vi "test json roundtrip.vi"(8 "error in (no error)":errorcluster, 11 "Enum":T1(ring)) -> (0 "error out":errorcluster, 1 "JSON out":string, 2 "JSON in":string, 3 "Passed?":bool, 5 "Result":variant)   [LabVIEW 2019, in "labview_json_tests.lvlib"]
uses:
  labview_json_tests.lvlib
  lib/labview_json.lvlib
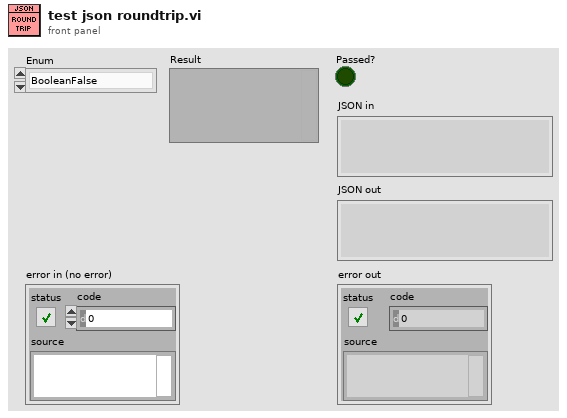
[diagram p1: front panel]
types:
  T1 = enum16{"BooleanFalse", "BooleanTrue", "StringSentence", "StringMultiline", "StringQuoted", "StringEscaped", "IntNumber", "IntMin", "IntMax", "IntI64", "IntI32", "IntI16", "IntI8", "UintNumber", "UintMin", "UintMax", "UintU64", "UintU32", "UintU16", "UintU8", "FloatNumber", "FloatMin", "FloatMax", "FloatZero", "FloatNaN", "FloatExt", "FloatDbl", "FloatSgl", "EnumU32", "EnumU16", "EnumU8", "EnumU32String", "EnumU16String", "EnumU8String", "EnumBadString", "PathAbs", "PathRel", "PathNetwork", "PathFile", "PathEmpty", "PathNaN", "PathCurrentDir", "PathParentDir", "TimeDateTime", "TimeDate", "NullVoid", "NullLVVariant", "NullBoolean", "NullInt", "NullUint", "NullFloat", "NullString", "NullPath", "NullEnum", "NullTime", "NullArray", "NullArrayVoid", "NullArrayLVVariant", "NullObject", "NullObjectVoid", "NullObjectLVVariant", "NullWaveform", "Array1DValues", "Array1DEmpty", "Array1DObject", "Array1DMulti", "Array2DValues", "Array2DEmpty", "Array3DValues", "Array3DEmpty", "ObjectValues", "ObjectEmpty", "ObjectWaveform", "ObjectReorder"}
  T2 = cluster{"I16":i16, "Bool":bool, "String":string, "Array":u32[]}
  T3 = enum16{"Item A", "Item B", "Item C", "Item D", "Item E"}
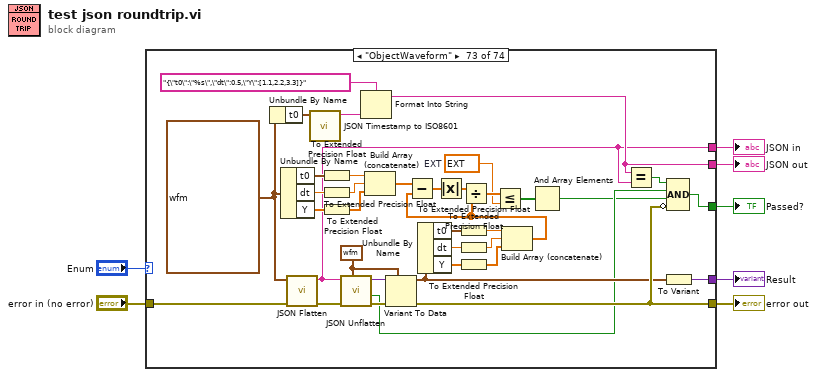
[diagram p0: block diagram]
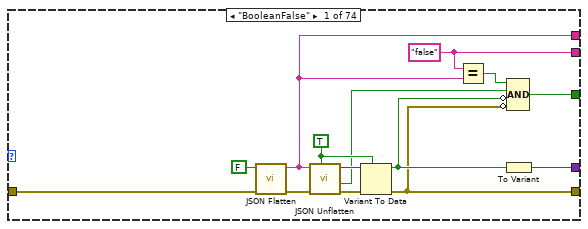
[diagram p2: hidden frame]
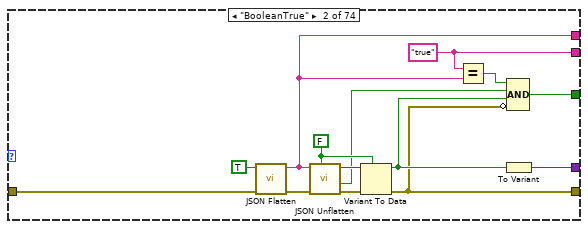
[diagram p3: hidden frame]
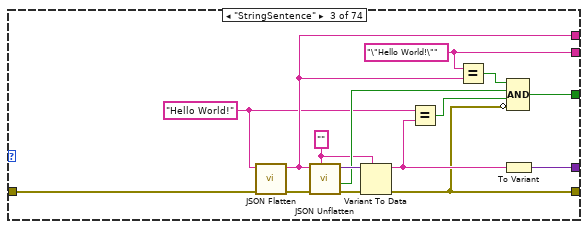
[diagram p4: hidden frame]
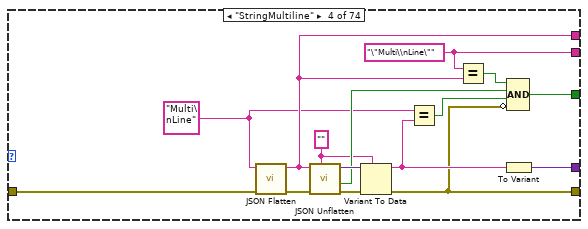
[diagram p5: hidden frame]
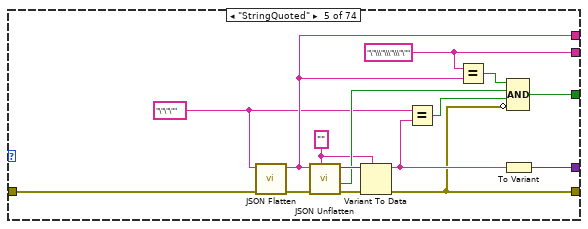
[diagram p6: hidden frame]
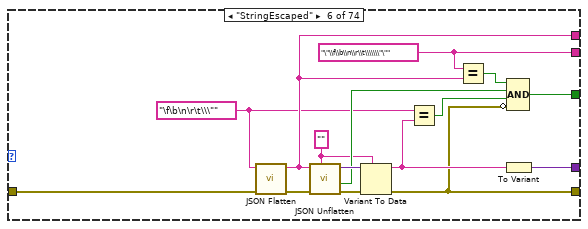
[diagram p7: hidden frame]
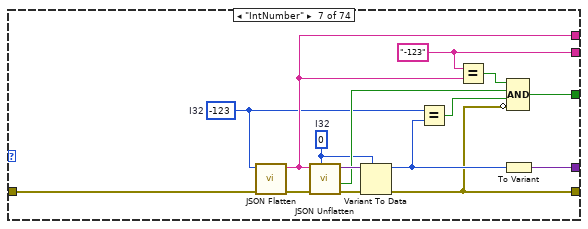
[diagram p8: hidden frame]
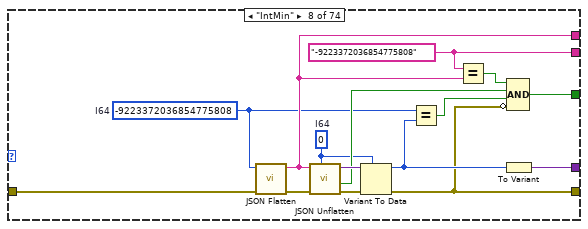
[diagram p9: hidden frame]
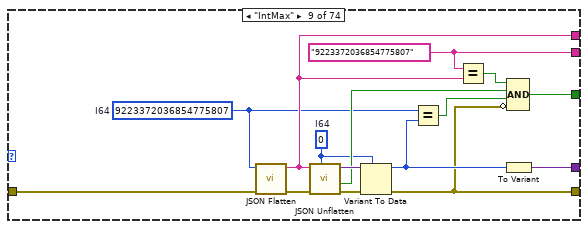
[diagram p10: hidden frame]
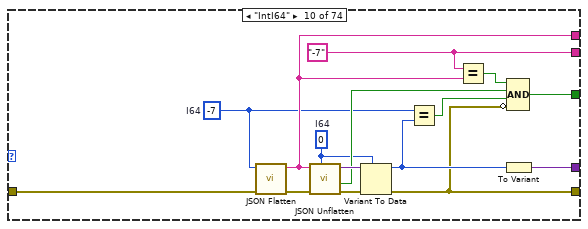
[diagram p11: hidden frame]
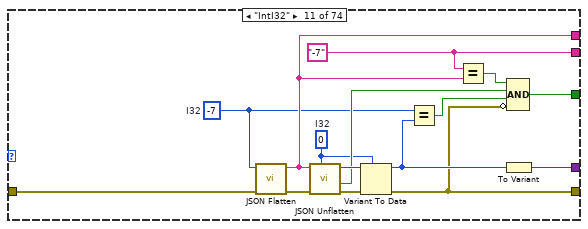
[diagram p12: hidden frame]
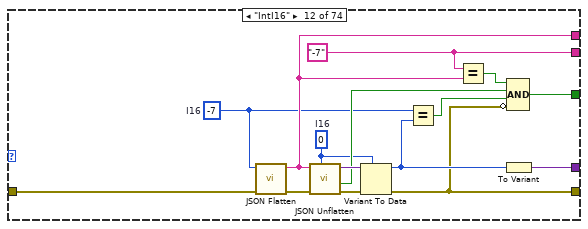
[diagram p13: hidden frame]
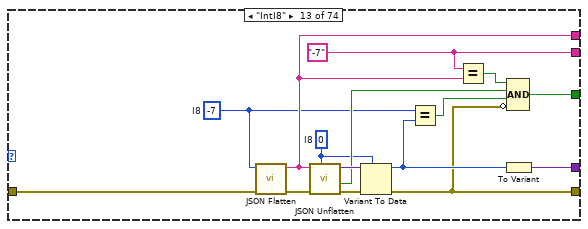
[diagram p14: hidden frame]
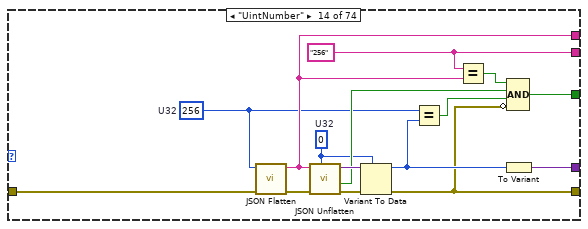
[diagram p15: hidden frame]
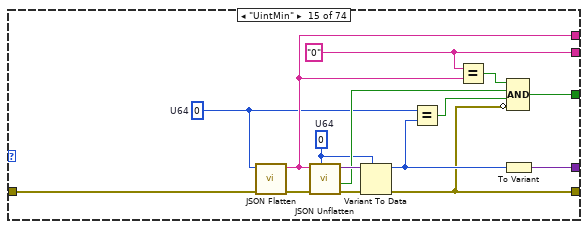
[diagram p16: hidden frame]
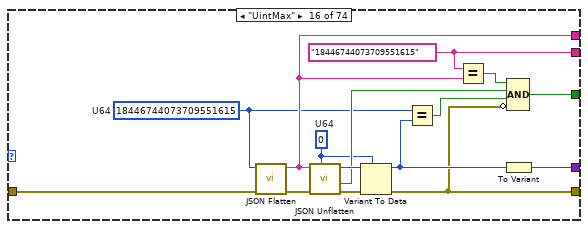
[diagram p17: hidden frame]
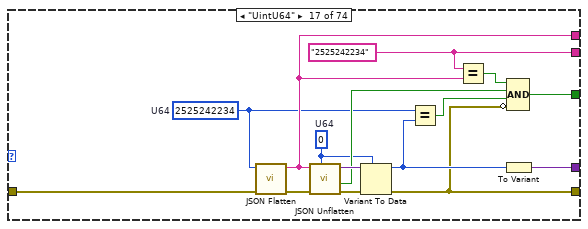
[diagram p18: hidden frame]
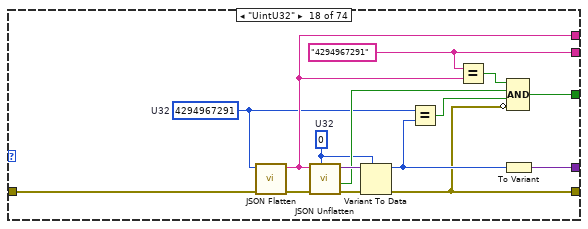
[diagram p19: hidden frame]
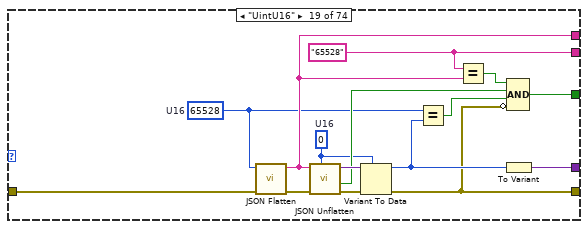
[diagram p20: hidden frame]
diagram:
  n1 = case shown="\"ObjectWaveform\"" "Enum" {
    tunnel: "error in (no error)" -> [w17 w31 w46 w61 w76 w91 w106 w121 w136 w151 w166 w181 w196 w211 w226 w241 w256 w271 w286 w301 w320 w335 w350 w365 w380 w399 w418 w437 w453 w469 w485 w501 w517 w533 w549 w564 w579 w594 w609 w624 w639 w654 w669 w694 w702 w731 w750 w758 w771 w784 w797 w810 w822 w835 w848 w862 w873 w887 w901 w914 w929 w942 w961 w977 w992 w1024 w1040 w1056 w1072 w1088 w1105 w1122 w1159 w1179]
    tunnel: [w8 w22 w36 w51 w66 w81 w96 w111 w126 w141 w156 w171 w186 w201 w216 w231 w246 w261 w276 w291 w306 w325 w340 w355 w370 w385 w404 w423 w442 w458 w474 w490 w506 w522 w539 w554 w569 w584 w599 w614 w629 w644 w659 w688 w713 w725 w740 w759 w772 w785 w798 w811 w823 w836 w849 w863 w875 w889 w902 w915 w930 w943 w951 w967 w986 w1019 w1030 w1046 w1062 w1078 w1099 w1116 w1156 w1173] -> w6
    tunnel: [w20 w34 w49 w64 w79 w94 w109 w124 w139 w154 w169 w184 w199 w214 w229 w244 w259 w274 w289 w304 w323 w338 w353 w368 w383 w402 w421 w440 w456 w472 w488 w504 w520 w536 w552 w567 w582 w597 w612 w627 w642 w657 w672 w697 w719 w734 w753 w764 w777 w790 w803 w816 w828 w841 w854 w868 w880 w894 w907 w920 w935 w948 w964 w980 w995 w1027 w1043 w1059 w1075 w1091 w1108 w1125 w1162 w1182] -> w5
    tunnel: [w19 w33 w48 w63 w78 w93 w108 w123 w138 w153 w168 w183 w198 w213 w228 w243 w258 w273 w288 w303 w322 w337 w352 w367 w382 w401 w420 w439 w455 w471 w487 w503 w519 w535 w551 w566 w581 w596 w611 w626 w641 w656 w671 w696 w718 w733 w752 w763 w776 w789 w802 w815 w827 w840 w853 w867 w879 w893 w906 w919 w934 w947 w963 w979 w994 w1026 w1042 w1058 w1074 w1090 w1107 w1124 w1161 w1181] -> w4
    tunnel: [w9 w23 w41 w56 w71 w82 w99 w114 w129 w144 w159 w174 w189 w204 w219 w234 w249 w264 w279 w294 w315 w330 w345 w360 w375 w394 w413 w432 w446 w462 w478 w494 w510 w526 w543 w557 w572 w587 w602 w617 w632 w647 w662 w676 w699 w728 w747 w755 w770 w783 w796 w809 w821 w834 w847 w861 w874 w888 w900 w913 w928 w941 w954 w970 w984 w1018 w1033 w1049 w1065 w1081 w1100 w1117 w1151 w1174] -> w2
    tunnel: [w15 w29 w44 w59 w74 w89 w104 w119 w134 w149 w164 w179 w194 w209 w224 w239 w254 w269 w284 w299 w318 w333 w348 w363 w378 w397 w416 w435 w451 w467 w483 w499 w515 w531 w547 w562 w577 w592 w607 w622 w637 w652 w667 w692 w699 w730 w749 w755 w770 w783 w796 w809 w821 w834 w847 w861 w874 w888 w900 w913 w928 w941 w959 w975 w990 w1022 w1038 w1054 w1070 w1086 w1103 w1120 w1132 w1177] -> w1
    frame "BooleanFalse" {
      w9 = "false"
      w12 = TRUE
      n2 = call "JSON Flatten.vi"("error in (no error)"=w17, "Variant in"=FALSE) -> ("error out"=w18:errorcluster, "JSON out"=w15:string)  [unwired: 8 in]
      n3 = call "JSON Unflatten.vi"("Variant Type"=w12, "error in (no error)"=w18, "JSON in"=w15) -> ("error out"=w16:errorcluster, "Exists?"=w11:bool, "Variant out"=w13:variant)  [unwired: 6 in]
      n4 = Variant To Data(error in=w16, type=w12, Variant=w13) -> (data=w10:bool, error out=w8:errorcluster)
      n5 = Equal?(x=w9, y=w15) -> (x = y?=w21:bool)
      n6 = To Variant(anything=w10) -> (Variant=w19:variant)
      n7 = Compound Arithmetic op=AND(w21, w11, invert w10, invert w8) -> (w20:bool)
    }
    frame "BooleanTrue" {
      w23 = "true"
      w26 = FALSE
      n8 = call "JSON Flatten.vi"("error in (no error)"=w31, "Variant in"=TRUE) -> ("error out"=w32:errorcluster, "JSON out"=w29:string)  [unwired: 8 in]
      n9 = call "JSON Unflatten.vi"("Variant Type"=w26, "error in (no error)"=w32, "JSON in"=w29) -> ("error out"=w30:errorcluster, "Exists?"=w25:bool, "Variant out"=w27:variant)  [unwired: 6 in]
      n10 = Variant To Data(error in=w30, type=w26, Variant=w27) -> (data=w24:bool, error out=w22:errorcluster)
      n11 = Equal?(x=w23, y=w29) -> (x = y?=w35:bool)
      n12 = To Variant(anything=w24) -> (Variant=w33:variant)
      n13 = Compound Arithmetic op=AND(w35, w25, w24, invert w22) -> (w34:bool)
    }
    frame "StringSentence" {
      w40 = ""
      w38 = "Hello World!"
      w41 = "\"Hello World!\""
      n14 = call "JSON Flatten.vi"("error in (no error)"=w46, "Variant in"=w38) -> ("error out"=w47:errorcluster, "JSON out"=w44:string)  [unwired: 8 in]
      n15 = call "JSON Unflatten.vi"("Variant Type"=w40, "error in (no error)"=w47, "JSON in"=w44) -> ("error out"=w45:errorcluster, "Exists?"=w42:bool, "Variant out"=w43:variant)  [unwired: 6 in]
      n16 = Variant To Data(error in=w45, type=w40, Variant=w43) -> (data=w39:string, error out=w36:errorcluster)
      n17 = Equal?(x=w38, y=w39) -> (x = y?=w37:bool)
      n18 = Equal?(x=w41, y=w44) -> (x = y?=w50:bool)
      n19 = To Variant(anything=w39) -> (Variant=w48:variant)
      n20 = Compound Arithmetic op=AND(w50, w42, w37, invert w36) -> (w49:bool)
    }
    frame "StringMultiline" {
      w55 = ""
      w53 = "Multi\nLine"
      w56 = "\"Multi\\nLine\""
      n21 = call "JSON Flatten.vi"("error in (no error)"=w61, "Variant in"=w53) -> ("error out"=w62:errorcluster, "JSON out"=w59:string)  [unwired: 8 in]
      n22 = call "JSON Unflatten.vi"("Variant Type"=w55, "error in (no error)"=w62, "JSON in"=w59) -> ("error out"=w60:errorcluster, "Exists?"=w57:bool, "Variant out"=w58:variant)  [unwired: 6 in]
      n23 = Variant To Data(error in=w60, type=w55, Variant=w58) -> (data=w54:string, error out=w51:errorcluster)
      n24 = Equal?(x=w53, y=w54) -> (x = y?=w52:bool)
      n25 = Equal?(x=w56, y=w59) -> (x = y?=w65:bool)
      n26 = To Variant(anything=w54) -> (Variant=w63:variant)
      n27 = Compound Arithmetic op=AND(w65, w57, w52, invert w51) -> (w64:bool)
    }
    frame "StringQuoted" {
      w70 = ""
      w68 = "\"\"\""
      w71 = "\"\\\"\\\"\\\"\""
      n28 = call "JSON Flatten.vi"("error in (no error)"=w76, "Variant in"=w68) -> ("error out"=w77:errorcluster, "JSON out"=w74:string)  [unwired: 8 in]
      n29 = call "JSON Unflatten.vi"("Variant Type"=w70, "error in (no error)"=w77, "JSON in"=w74) -> ("error out"=w75:errorcluster, "Exists?"=w72:bool, "Variant out"=w73:variant)  [unwired: 6 in]
      n30 = Variant To Data(error in=w75, type=w70, Variant=w73) -> (data=w69:string, error out=w66:errorcluster)
      n31 = Equal?(x=w68, y=w69) -> (x = y?=w67:bool)
      n32 = Equal?(x=w71, y=w74) -> (x = y?=w80:bool)
      n33 = To Variant(anything=w69) -> (Variant=w78:variant)
      n34 = Compound Arithmetic op=AND(w80, w72, w67, invert w66) -> (w79:bool)
    }
    frame "StringEscaped" {
      w83 = "\f\b\n\r\t\\\""
      w82 = "\"\\f\\b\\n\\r\\t\\\\\\\"\""
      w86 = ""
      n35 = call "JSON Flatten.vi"("error in (no error)"=w91, "Variant in"=w83) -> ("error out"=w92:errorcluster, "JSON out"=w89:string)  [unwired: 8 in]
      n36 = call "JSON Unflatten.vi"("Variant Type"=w86, "error in (no error)"=w92, "JSON in"=w89) -> ("error out"=w90:errorcluster, "Exists?"=w87:bool, "Variant out"=w88:variant)  [unwired: 6 in]
      n37 = Variant To Data(error in=w90, type=w86, Variant=w88) -> (data=w85:string, error out=w81:errorcluster)
      n38 = Equal?(x=w83, y=w85) -> (x = y?=w84:bool)
      n39 = Equal?(x=w82, y=w89) -> (x = y?=w95:bool)
      n40 = To Variant(anything=w85) -> (Variant=w93:variant)
      n41 = Compound Arithmetic op=AND(w95, w87, w84, invert w81) -> (w94:bool)
    }
    frame "IntNumber" {
      w97 = 0  # I32
      w98 = -123  # I32
      w99 = "-123"
      n42 = call "JSON Flatten.vi"("error in (no error)"=w106, "Variant in"=w98) -> ("error out"=w107:errorcluster, "JSON out"=w104:string)  [unwired: 8 in]
      n43 = call "JSON Unflatten.vi"("Variant Type"=w97, "error in (no error)"=w107, "JSON in"=w104) -> ("error out"=w105:errorcluster, "Exists?"=w102:bool, "Variant out"=w103:variant)  [unwired: 6 in]
      n44 = Variant To Data(error in=w105, type=w97, Variant=w103) -> (data=w101:i32, error out=w96:errorcluster)
      n45 = Equal?(x=w98, y=w101) -> (x = y?=w100:bool)
      n46 = Equal?(x=w99, y=w104) -> (x = y?=w110:bool)
      n47 = To Variant(anything=w101) -> (Variant=w108:variant)
      n48 = Compound Arithmetic op=AND(w110, w102, w100, invert w96) -> (w109:bool)
    }
    frame "IntMin" {
      w112 = i64 0  # I64
      w113 = i64 -9223372036854775808  # I64
      w114 = "-9223372036854775808"
      n49 = call "JSON Flatten.vi"("error in (no error)"=w121, "Variant in"=w113) -> ("error out"=w122:errorcluster, "JSON out"=w119:string)  [unwired: 8 in]
      n50 = call "JSON Unflatten.vi"("Variant Type"=w112, "error in (no error)"=w122, "JSON in"=w119) -> ("error out"=w120:errorcluster, "Exists?"=w117:bool, "Variant out"=w118:variant)  [unwired: 6 in]
      n51 = Variant To Data(error in=w120, type=w112, Variant=w118) -> (data=w116:i64, error out=w111:errorcluster)
      n52 = Equal?(x=w113, y=w116) -> (x = y?=w115:bool)
      n53 = Equal?(x=w114, y=w119) -> (x = y?=w125:bool)
      n54 = To Variant(anything=w116) -> (Variant=w123:variant)
      n55 = Compound Arithmetic op=AND(w125, w117, w115, invert w111) -> (w124:bool)
    }
    frame "IntMax" {
      w127 = i64 0  # I64
      w128 = i64 9223372036854775807  # I64
      w129 = "9223372036854775807"
      n56 = call "JSON Flatten.vi"("error in (no error)"=w136, "Variant in"=w128) -> ("error out"=w137:errorcluster, "JSON out"=w134:string)  [unwired: 8 in]
      n57 = call "JSON Unflatten.vi"("Variant Type"=w127, "error in (no error)"=w137, "JSON in"=w134) -> ("error out"=w135:errorcluster, "Exists?"=w132:bool, "Variant out"=w133:variant)  [unwired: 6 in]
      n58 = Variant To Data(error in=w135, type=w127, Variant=w133) -> (data=w131:i64, error out=w126:errorcluster)
      n59 = Equal?(x=w128, y=w131) -> (x = y?=w130:bool)
      n60 = Equal?(x=w129, y=w134) -> (x = y?=w140:bool)
      n61 = To Variant(anything=w131) -> (Variant=w138:variant)
      n62 = Compound Arithmetic op=AND(w140, w132, w130, invert w126) -> (w139:bool)
    }
    frame "IntI64" {
      w142 = i64 0  # I64
      w143 = i64 -7  # I64
      w144 = "-7"
      n63 = call "JSON Flatten.vi"("error in (no error)"=w151, "Variant in"=w143) -> ("error out"=w152:errorcluster, "JSON out"=w149:string)  [unwired: 8 in]
      n64 = call "JSON Unflatten.vi"("Variant Type"=w142, "error in (no error)"=w152, "JSON in"=w149) -> ("error out"=w150:errorcluster, "Exists?"=w147:bool, "Variant out"=w148:variant)  [unwired: 6 in]
      n65 = Variant To Data(error in=w150, type=w142, Variant=w148) -> (data=w146:i64, error out=w141:errorcluster)
      n66 = Equal?(x=w143, y=w146) -> (x = y?=w145:bool)
      n67 = Equal?(x=w144, y=w149) -> (x = y?=w155:bool)
      n68 = To Variant(anything=w146) -> (Variant=w153:variant)
      n69 = Compound Arithmetic op=AND(w155, w147, w145, invert w141) -> (w154:bool)
    }
    frame "IntI32" {
      w157 = 0  # I32
      w158 = -7  # I32
      w159 = "-7"
      n70 = call "JSON Flatten.vi"("error in (no error)"=w166, "Variant in"=w158) -> ("error out"=w167:errorcluster, "JSON out"=w164:string)  [unwired: 8 in]
      n71 = call "JSON Unflatten.vi"("Variant Type"=w157, "error in (no error)"=w167, "JSON in"=w164) -> ("error out"=w165:errorcluster, "Exists?"=w162:bool, "Variant out"=w163:variant)  [unwired: 6 in]
      n72 = Variant To Data(error in=w165, type=w157, Variant=w163) -> (data=w161:i32, error out=w156:errorcluster)
      n73 = Equal?(x=w158, y=w161) -> (x = y?=w160:bool)
      n74 = Equal?(x=w159, y=w164) -> (x = y?=w170:bool)
      n75 = To Variant(anything=w161) -> (Variant=w168:variant)
      n76 = Compound Arithmetic op=AND(w170, w162, w160, invert w156) -> (w169:bool)
    }
    frame "IntI16" {
      w172 = i16 0  # I16
      w173 = i16 -7  # I16
      w174 = "-7"
      n77 = call "JSON Flatten.vi"("error in (no error)"=w181, "Variant in"=w173) -> ("error out"=w182:errorcluster, "JSON out"=w179:string)  [unwired: 8 in]
      n78 = call "JSON Unflatten.vi"("Variant Type"=w172, "error in (no error)"=w182, "JSON in"=w179) -> ("error out"=w180:errorcluster, "Exists?"=w177:bool, "Variant out"=w178:variant)  [unwired: 6 in]
      n79 = Variant To Data(error in=w180, type=w172, Variant=w178) -> (data=w176:i16, error out=w171:errorcluster)
      n80 = Equal?(x=w173, y=w176) -> (x = y?=w175:bool)
      n81 = Equal?(x=w174, y=w179) -> (x = y?=w185:bool)
      n82 = To Variant(anything=w176) -> (Variant=w183:variant)
      n83 = Compound Arithmetic op=AND(w185, w177, w175, invert w171) -> (w184:bool)
    }
    frame "IntI8" {
      w187 = i8 0  # I8
      w188 = i8 -7  # I8
      w189 = "-7"
      n84 = call "JSON Flatten.vi"("error in (no error)"=w196, "Variant in"=w188) -> ("error out"=w197:errorcluster, "JSON out"=w194:string)  [unwired: 8 in]
      n85 = call "JSON Unflatten.vi"("Variant Type"=w187, "error in (no error)"=w197, "JSON in"=w194) -> ("error out"=w195:errorcluster, "Exists?"=w192:bool, "Variant out"=w193:variant)  [unwired: 6 in]
      n86 = Variant To Data(error in=w195, type=w187, Variant=w193) -> (data=w191:i8, error out=w186:errorcluster)
      n87 = Equal?(x=w188, y=w191) -> (x = y?=w190:bool)
      n88 = Equal?(x=w189, y=w194) -> (x = y?=w200:bool)
      n89 = To Variant(anything=w191) -> (Variant=w198:variant)
      n90 = Compound Arithmetic op=AND(w200, w192, w190, invert w186) -> (w199:bool)
    }
    frame "UintNumber" {
      w202 = u32 0  # U32
      w203 = u32 256  # U32
      w204 = "256"
      n91 = call "JSON Flatten.vi"("error in (no error)"=w211, "Variant in"=w203) -> ("error out"=w212:errorcluster, "JSON out"=w209:string)  [unwired: 8 in]
      n92 = call "JSON Unflatten.vi"("Variant Type"=w202, "error in (no error)"=w212, "JSON in"=w209) -> ("error out"=w210:errorcluster, "Exists?"=w207:bool, "Variant out"=w208:variant)  [unwired: 6 in]
      n93 = Variant To Data(error in=w210, type=w202, Variant=w208) -> (data=w206:u32, error out=w201:errorcluster)
      n94 = Equal?(x=w203, y=w206) -> (x = y?=w205:bool)
      n95 = Equal?(x=w204, y=w209) -> (x = y?=w215:bool)
      n96 = To Variant(anything=w206) -> (Variant=w213:variant)
      n97 = Compound Arithmetic op=AND(w215, w207, w205, invert w201) -> (w214:bool)
    }
    frame "UintMin" {
      w217 = u64 0  # U64
      w218 = u64 0  # U64
      w219 = "0"
      n98 = call "JSON Flatten.vi"("error in (no error)"=w226, "Variant in"=w218) -> ("error out"=w227:errorcluster, "JSON out"=w224:string)  [unwired: 8 in]
      n99 = call "JSON Unflatten.vi"("Variant Type"=w217, "error in (no error)"=w227, "JSON in"=w224) -> ("error out"=w225:errorcluster, "Exists?"=w222:bool, "Variant out"=w223:variant)  [unwired: 6 in]
      n100 = Variant To Data(error in=w225, type=w217, Variant=w223) -> (data=w221:u64, error out=w216:errorcluster)
      n101 = Equal?(x=w218, y=w221) -> (x = y?=w220:bool)
      n102 = Equal?(x=w219, y=w224) -> (x = y?=w230:bool)
      n103 = To Variant(anything=w221) -> (Variant=w228:variant)
      n104 = Compound Arithmetic op=AND(w230, w222, w220, invert w216) -> (w229:bool)
    }
    frame "UintMax" {
      w232 = u64 0  # U64
      w233 = u64 18446744073709551615  # U64
      w234 = "18446744073709551615"
      n105 = call "JSON Flatten.vi"("error in (no error)"=w241, "Variant in"=w233) -> ("error out"=w242:errorcluster, "JSON out"=w239:string)  [unwired: 8 in]
      n106 = call "JSON Unflatten.vi"("Variant Type"=w232, "error in (no error)"=w242, "JSON in"=w239) -> ("error out"=w240:errorcluster, "Exists?"=w237:bool, "Variant out"=w238:variant)  [unwired: 6 in]
      n107 = Variant To Data(error in=w240, type=w232, Variant=w238) -> (data=w236:u64, error out=w231:errorcluster)
      n108 = Equal?(x=w233, y=w236) -> (x = y?=w235:bool)
      n109 = Equal?(x=w234, y=w239) -> (x = y?=w245:bool)
      n110 = To Variant(anything=w236) -> (Variant=w243:variant)
      n111 = Compound Arithmetic op=AND(w245, w237, w235, invert w231) -> (w244:bool)
    }
    frame "UintU64" {
      w247 = u64 0  # U64
      w248 = u64 2525242234  # U64
      w249 = "2525242234"
      n112 = call "JSON Flatten.vi"("error in (no error)"=w256, "Variant in"=w248) -> ("error out"=w257:errorcluster, "JSON out"=w254:string)  [unwired: 8 in]
      n113 = call "JSON Unflatten.vi"("Variant Type"=w247, "error in (no error)"=w257, "JSON in"=w254) -> ("error out"=w255:errorcluster, "Exists?"=w252:bool, "Variant out"=w253:variant)  [unwired: 6 in]
      n114 = Variant To Data(error in=w255, type=w247, Variant=w253) -> (data=w251:u64, error out=w246:errorcluster)
      n115 = Equal?(x=w248, y=w251) -> (x = y?=w250:bool)
      n116 = Equal?(x=w249, y=w254) -> (x = y?=w260:bool)
      n117 = To Variant(anything=w251) -> (Variant=w258:variant)
      n118 = Compound Arithmetic op=AND(w260, w252, w250, invert w246) -> (w259:bool)
    }
    frame "UintU32" {
      w262 = u32 0  # U32
      w263 = u32 4294967291  # U32
      w264 = "4294967291"
      n119 = call "JSON Flatten.vi"("error in (no error)"=w271, "Variant in"=w263) -> ("error out"=w272:errorcluster, "JSON out"=w269:string)  [unwired: 8 in]
      n120 = call "JSON Unflatten.vi"("Variant Type"=w262, "error in (no error)"=w272, "JSON in"=w269) -> ("error out"=w270:errorcluster, "Exists?"=w267:bool, "Variant out"=w268:variant)  [unwired: 6 in]
      n121 = Variant To Data(error in=w270, type=w262, Variant=w268) -> (data=w266:u32, error out=w261:errorcluster)
      n122 = Equal?(x=w263, y=w266) -> (x = y?=w265:bool)
      n123 = Equal?(x=w264, y=w269) -> (x = y?=w275:bool)
      n124 = To Variant(anything=w266) -> (Variant=w273:variant)
      n125 = Compound Arithmetic op=AND(w275, w267, w265, invert w261) -> (w274:bool)
    }
    frame "UintU16" {
      w277 = u16 0  # U16
      w278 = u16 65528  # U16
      w279 = "65528"
      n126 = call "JSON Flatten.vi"("error in (no error)"=w286, "Variant in"=w278) -> ("error out"=w287:errorcluster, "JSON out"=w284:string)  [unwired: 8 in]
      n127 = call "JSON Unflatten.vi"("Variant Type"=w277, "error in (no error)"=w287, "JSON in"=w284) -> ("error out"=w285:errorcluster, "Exists?"=w282:bool, "Variant out"=w283:variant)  [unwired: 6 in]
      n128 = Variant To Data(error in=w285, type=w277, Variant=w283) -> (data=w281:u16, error out=w276:errorcluster)
      n129 = Equal?(x=w278, y=w281) -> (x = y?=w280:bool)
      n130 = Equal?(x=w279, y=w284) -> (x = y?=w290:bool)
      n131 = To Variant(anything=w281) -> (Variant=w288:variant)
      n132 = Compound Arithmetic op=AND(w290, w282, w280, invert w276) -> (w289:bool)
    }
    frame "UintU8" {
      w292 = u8 0  # U8
      w293 = u8 248  # U8
      w294 = "248"
      n133 = call "JSON Flatten.vi"("error in (no error)"=w301, "Variant in"=w293) -> ("error out"=w302:errorcluster, "JSON out"=w299:string)  [unwired: 8 in]
      n134 = call "JSON Unflatten.vi"("Variant Type"=w292, "error in (no error)"=w302, "JSON in"=w299) -> ("error out"=w300:errorcluster, "Exists?"=w297:bool, "Variant out"=w298:variant)  [unwired: 6 in]
      n135 = Variant To Data(error in=w300, type=w292, Variant=w298) -> (data=w296:u8, error out=w291:errorcluster)
      n136 = Equal?(x=w293, y=w296) -> (x = y?=w295:bool)
      n137 = Equal?(x=w294, y=w299) -> (x = y?=w305:bool)
      n138 = To Variant(anything=w296) -> (Variant=w303:variant)
      n139 = Compound Arithmetic op=AND(w305, w297, w295, invert w291) -> (w304:bool)
    }
    frame "FloatNumber" {
      w314 = 0.0  # DBL
      w313 = -42949.67289234  # DBL
      w315 = "-42949.67289234"
      n140 = call "JSON Flatten.vi"("error in (no error)"=w320, "Variant in"=w313) -> ("error out"=w321:errorcluster, "JSON out"=w318:string)  [unwired: 8 in]
      n141 = call "JSON Unflatten.vi"("Variant Type"=w314, "error in (no error)"=w321, "JSON in"=w318) -> ("error out"=w319:errorcluster, "Exists?"=w316:bool, "Variant out"=w317:variant)  [unwired: 6 in]
      n142 = Variant To Data(error in=w319, type=w314, Variant=w317) -> (data=w310:dbl, error out=w306:errorcluster)
      n143 = Subtract(x=w313, y=w310) -> (x-y=w312:dbl)
      n144 = Absolute Value(x=w312) -> (abs(x)=w311:dbl)
      n145 = Divide(x=w311, y=w310) -> (x/y=w309:dbl)
      n146 = Equal?(x=w315, y=w318) -> (x = y?=w324:bool)
      n147 = Less Or Equal?(x=w309, y=1e-11) -> (x <= y?=w307:bool)
      n148 = To Variant(anything=w310) -> (Variant=w322:variant)
      n149 = Compound Arithmetic op=AND(w324, w316, w307, invert w306) -> (w323:bool)
    }
    frame "FloatMin" {
      w329 = 0.0  # DBL
      w328 = -inf  # DBL
      w330 = "-Infinity"
      n150 = call "JSON Flatten.vi"("error in (no error)"=w335, "Variant in"=w328) -> ("error out"=w336:errorcluster, "JSON out"=w333:string)  [unwired: 8 in]
      n151 = call "JSON Unflatten.vi"("Variant Type"=w329, "error in (no error)"=w336, "JSON in"=w333) -> ("error out"=w334:errorcluster, "Exists?"=w331:bool, "Variant out"=w332:variant)  [unwired: 6 in]
      n152 = Variant To Data(error in=w334, type=w329, Variant=w332) -> (data=w327:dbl, error out=w325:errorcluster)
      n153 = Equal?(x=w330, y=w333) -> (x = y?=w339:bool)
      n154 = Equal?(x=w328, y=w327) -> (x = y?=w326:bool)
      n155 = To Variant(anything=w327) -> (Variant=w337:variant)
      n156 = Compound Arithmetic op=AND(w339, w331, w326, invert w325) -> (w338:bool)
    }
    frame "FloatMax" {
      w344 = 0.0  # DBL
      w343 = inf  # DBL
      w345 = "Infinity"
      n157 = call "JSON Flatten.vi"("error in (no error)"=w350, "Variant in"=w343) -> ("error out"=w351:errorcluster, "JSON out"=w348:string)  [unwired: 8 in]
      n158 = call "JSON Unflatten.vi"("Variant Type"=w344, "error in (no error)"=w351, "JSON in"=w348) -> ("error out"=w349:errorcluster, "Exists?"=w346:bool, "Variant out"=w347:variant)  [unwired: 6 in]
      n159 = Variant To Data(error in=w349, type=w344, Variant=w347) -> (data=w342:dbl, error out=w340:errorcluster)
      n160 = Equal?(x=w345, y=w348) -> (x = y?=w354:bool)
      n161 = Equal?(x=w343, y=w342) -> (x = y?=w341:bool)
      n162 = To Variant(anything=w342) -> (Variant=w352:variant)
      n163 = Compound Arithmetic op=AND(w354, w346, w341, invert w340) -> (w353:bool)
    }
    frame "FloatZero" {
      w359 = 2.0  # DBL
      w358 = 0.0  # DBL
      w360 = "0"
      n164 = call "JSON Flatten.vi"("error in (no error)"=w365, "Variant in"=w358) -> ("error out"=w366:errorcluster, "JSON out"=w363:string)  [unwired: 8 in]
      n165 = call "JSON Unflatten.vi"("Variant Type"=w359, "error in (no error)"=w366, "JSON in"=w363) -> ("error out"=w364:errorcluster, "Exists?"=w361:bool, "Variant out"=w362:variant)  [unwired: 6 in]
      n166 = Variant To Data(error in=w364, type=w359, Variant=w362) -> (data=w357:dbl, error out=w355:errorcluster)
      n167 = Equal?(x=w360, y=w363) -> (x = y?=w369:bool)
      n168 = Equal?(x=w358, y=w357) -> (x = y?=w356:bool)
      n169 = To Variant(anything=w357) -> (Variant=w367:variant)
      n170 = Compound Arithmetic op=AND(w369, w361, w356, invert w355) -> (w368:bool)
    }
    frame "FloatNaN" {
      w374 = 2.0  # DBL
      w373 = nan  # DBL
      w375 = "NaN"
      n171 = call "JSON Flatten.vi"("error in (no error)"=w380, "Variant in"=w373) -> ("error out"=w381:errorcluster, "JSON out"=w378:string)  [unwired: 8 in]
      n172 = call "JSON Unflatten.vi"("Variant Type"=w374, "error in (no error)"=w381, "JSON in"=w378) -> ("error out"=w379:errorcluster, "Exists?"=w376:bool, "Variant out"=w377:variant)  [unwired: 6 in]
      n173 = Variant To Data(error in=w379, type=w374, Variant=w377) -> (data=w372:dbl, error out=w370:errorcluster)
      n174 = Not A Number/Path/Refnum?(number/path/refnum=w372) -> (NaN/Path/Refnum?=w371:bool)
      n175 = Equal?(x=w375, y=w378) -> (x = y?=w384:bool)
      n176 = To Variant(anything=w372) -> (Variant=w382:variant)
      n177 = Compound Arithmetic op=AND(w384, w376, w371, invert w370) -> (w383:bool)
    }
    frame "FloatExt" {
      w387 = ext 1e-13  # EXT
      w393 = ext 0.0  # EXT
      w392 = ext 1.844674407371e+19  # EXT
      w394 = "1.844674407371E+19"
      n178 = call "JSON Flatten.vi"("error in (no error)"=w399, "Variant in"=w392) -> ("error out"=w400:errorcluster, "JSON out"=w397:string)  [unwired: 8 in]
      n179 = call "JSON Unflatten.vi"("Variant Type"=w393, "error in (no error)"=w400, "JSON in"=w397) -> ("error out"=w398:errorcluster, "Exists?"=w395:bool, "Variant out"=w396:variant)  [unwired: 6 in]
      n180 = Variant To Data(error in=w398, type=w393, Variant=w396) -> (data=w389:ext, error out=w385:errorcluster)
      n181 = Subtract(x=w392, y=w389) -> (x-y=w391:ext)
      n182 = Absolute Value(x=w391) -> (abs(x)=w390:ext)
      n183 = Divide(x=w390, y=w389) -> (x/y=w388:ext)
      n184 = Equal?(x=w394, y=w397) -> (x = y?=w403:bool)
      n185 = Less Or Equal?(x=w388, y=w387) -> (x <= y?=w386:bool)
      n186 = To Variant(anything=w389) -> (Variant=w401:variant)
      n187 = Compound Arithmetic op=AND(w403, w395, w386, invert w385) -> (w402:bool)
    }
    frame "FloatDbl" {
      w406 = 1e-11  # DBL
      w412 = 0.0  # DBL
      w411 = -19273791.23844  # DBL
      w413 = "-19273791.2384399995"
      n188 = call "JSON Flatten.vi"("error in (no error)"=w418, "Variant in"=w411) -> ("error out"=w419:errorcluster, "JSON out"=w416:string)  [unwired: 8 in]
      n189 = call "JSON Unflatten.vi"("Variant Type"=w412, "error in (no error)"=w419, "JSON in"=w416) -> ("error out"=w417:errorcluster, "Exists?"=w414:bool, "Variant out"=w415:variant)  [unwired: 6 in]
      n190 = Variant To Data(error in=w417, type=w412, Variant=w415) -> (data=w408:dbl, error out=w404:errorcluster)
      n191 = Subtract(x=w411, y=w408) -> (x-y=w410:dbl)
      n192 = Absolute Value(x=w410) -> (abs(x)=w409:dbl)
      n193 = Divide(x=w409, y=w408) -> (x/y=w407:dbl)
      n194 = Equal?(x=w413, y=w416) -> (x = y?=w422:bool)
      n195 = Less Or Equal?(x=w407, y=w406) -> (x <= y?=w405:bool)
      n196 = To Variant(anything=w408) -> (Variant=w420:variant)
      n197 = Compound Arithmetic op=AND(w422, w414, w405, invert w404) -> (w421:bool)
    }
    frame "FloatSgl" {
      w425 = sgl 1e-05  # SGL
      w431 = sgl 0.0  # SGL
      w430 = sgl 82833.23  # SGL
      w432 = "82833.2265625"
      n198 = call "JSON Flatten.vi"("error in (no error)"=w437, "Variant in"=w430) -> ("error out"=w438:errorcluster, "JSON out"=w435:string)  [unwired: 8 in]
      n199 = call "JSON Unflatten.vi"("Variant Type"=w431, "error in (no error)"=w438, "JSON in"=w435) -> ("error out"=w436:errorcluster, "Exists?"=w433:bool, "Variant out"=w434:variant)  [unwired: 6 in]
      n200 = Variant To Data(error in=w436, type=w431, Variant=w434) -> (data=w427:sgl, error out=w423:errorcluster)
      n201 = Subtract(x=w430, y=w427) -> (x-y=w429:sgl)
      n202 = Absolute Value(x=w429) -> (abs(x)=w428:sgl)
      n203 = Divide(x=w428, y=w427) -> (x/y=w426:sgl)
      n204 = Equal?(x=w432, y=w435) -> (x = y?=w441:bool)
      n205 = Less Or Equal?(x=w426, y=w425) -> (x <= y?=w424:bool)
      n206 = To Variant(anything=w427) -> (Variant=w439:variant)
      n207 = Compound Arithmetic op=AND(w441, w433, w424, invert w423) -> (w440:bool)
    }
    frame "EnumU32" {
      w444 = enum32{"Item A", "Item B", "Item C", "Item D"}."Item A"  # U32
      w445 = enum32{"Item A", "Item B", "Item C", "Item D"}."Item C"  # U32
      w446 = "2"
      n208 = call "JSON Flatten.vi"("Enums as string? (F)"=FALSE, "error in (no error)"=w453, "Variant in"=w445) -> ("error out"=w454:errorcluster, "JSON out"=w451:string)  [unwired: 7 in]
      n209 = call "JSON Unflatten.vi"("Variant Type"=w444, "error in (no error)"=w454, "JSON in"=w451) -> ("error out"=w452:errorcluster, "Exists?"=w449:bool, "Variant out"=w450:variant)  [unwired: 6 in]
      n210 = Variant To Data(error in=w452, type=w444, Variant=w450) -> (data=w448:enum32{"Item A", "Item B", "Item C", "Item D"}, error out=w442:errorcluster)
      n211 = Equal?(x=w445, y=w448) -> (x = y?=w447:bool)
      n212 = Equal?(x=w446, y=w451) -> (x = y?=w457:bool)
      n213 = To Variant(anything=w448) -> (Variant=w455:variant)
      n214 = Compound Arithmetic op=AND(w457, w449, w447, invert w442) -> (w456:bool)
    }
    frame "EnumU16" {
      w460 = enum16{"Item A", "Item B", "Item C", "Item D"}."Item A"  # U16
      w461 = enum16{"Item A", "Item B", "Item C", "Item D"}."Item B"  # U16
      w462 = "1"
      n215 = call "JSON Flatten.vi"("Enums as string? (F)"=FALSE, "error in (no error)"=w469, "Variant in"=w461) -> ("error out"=w470:errorcluster, "JSON out"=w467:string)  [unwired: 7 in]
      n216 = call "JSON Unflatten.vi"("Variant Type"=w460, "error in (no error)"=w470, "JSON in"=w467) -> ("error out"=w468:errorcluster, "Exists?"=w465:bool, "Variant out"=w466:variant)  [unwired: 6 in]
      n217 = Variant To Data(error in=w468, type=w460, Variant=w466) -> (data=w464:enum16{"Item A", "Item B", "Item C", "Item D"}, error out=w458:errorcluster)
      n218 = Equal?(x=w461, y=w464) -> (x = y?=w463:bool)
      n219 = Equal?(x=w462, y=w467) -> (x = y?=w473:bool)
      n220 = To Variant(anything=w464) -> (Variant=w471:variant)
      n221 = Compound Arithmetic op=AND(w473, w465, w463, invert w458) -> (w472:bool)
    }
    frame "EnumU8" {
      w476 = enum8{"Item A", "Item B", "Item C", "Item D"}."Item A"  # U8
      w477 = enum8{"Item A", "Item B", "Item C", "Item D"}."Item C"  # U8
      w478 = "2"
      n222 = call "JSON Flatten.vi"("Enums as string? (F)"=FALSE, "error in (no error)"=w485, "Variant in"=w477) -> ("error out"=w486:errorcluster, "JSON out"=w483:string)  [unwired: 7 in]
      n223 = call "JSON Unflatten.vi"("Variant Type"=w476, "error in (no error)"=w486, "JSON in"=w483) -> ("error out"=w484:errorcluster, "Exists?"=w481:bool, "Variant out"=w482:variant)  [unwired: 6 in]
      n224 = Variant To Data(error in=w484, type=w476, Variant=w482) -> (data=w480:enum8{"Item A", "Item B", "Item C", "Item D"}, error out=w474:errorcluster)
      n225 = Equal?(x=w477, y=w480) -> (x = y?=w479:bool)
      n226 = Equal?(x=w478, y=w483) -> (x = y?=w489:bool)
      n227 = To Variant(anything=w480) -> (Variant=w487:variant)
      n228 = Compound Arithmetic op=AND(w489, w481, w479, invert w474) -> (w488:bool)
    }
    frame "EnumU32String" {
      w492 = enum32{"Item A", "Item B", "Item C", "Item D"}."Item A"  # U32
      w493 = enum32{"Item A", "Item B", "Item C", "Item D"}."Item C"  # U32
      w494 = "\"Item C\""
      n229 = call "JSON Flatten.vi"("Enums as string? (F)"=TRUE, "error in (no error)"=w501, "Variant in"=w493) -> ("error out"=w502:errorcluster, "JSON out"=w499:string)  [unwired: 7 in]
      n230 = call "JSON Unflatten.vi"("Variant Type"=w492, "error in (no error)"=w502, "JSON in"=w499) -> ("error out"=w500:errorcluster, "Exists?"=w497:bool, "Variant out"=w498:variant)  [unwired: 6 in]
      n231 = Variant To Data(error in=w500, type=w492, Variant=w498) -> (data=w496:enum32{"Item A", "Item B", "Item C", "Item D"}, error out=w490:errorcluster)
      n232 = Equal?(x=w493, y=w496) -> (x = y?=w495:bool)
      n233 = Equal?(x=w494, y=w499) -> (x = y?=w505:bool)
      n234 = To Variant(anything=w496) -> (Variant=w503:variant)
      n235 = Compound Arithmetic op=AND(w505, w497, w495, invert w490) -> (w504:bool)
    }
    frame "EnumU16String" {
      w508 = enum16{"Item A", "Item B", "Item C", "Item D"}."Item A"  # U16
      w509 = enum16{"Item A", "Item B", "Item C", "Item D"}."Item B"  # U16
      w510 = "\"Item B\""
      n236 = call "JSON Flatten.vi"("Enums as string? (F)"=TRUE, "error in (no error)"=w517, "Variant in"=w509) -> ("error out"=w518:errorcluster, "JSON out"=w515:string)  [unwired: 7 in]
      n237 = call "JSON Unflatten.vi"("Variant Type"=w508, "error in (no error)"=w518, "JSON in"=w515) -> ("error out"=w516:errorcluster, "Exists?"=w513:bool, "Variant out"=w514:variant)  [unwired: 6 in]
      n238 = Variant To Data(error in=w516, type=w508, Variant=w514) -> (data=w512:enum16{"Item A", "Item B", "Item C", "Item D"}, error out=w506:errorcluster)
      n239 = Equal?(x=w509, y=w512) -> (x = y?=w511:bool)
      n240 = Equal?(x=w510, y=w515) -> (x = y?=w521:bool)
      n241 = To Variant(anything=w512) -> (Variant=w519:variant)
      n242 = Compound Arithmetic op=AND(w521, w513, w511, invert w506) -> (w520:bool)
    }
    frame "EnumU8String" {
      w524 = enum8{"Item A", "Item B", "Item C", "Item D"}."Item A"  # U8
      w525 = enum8{"Item A", "Item B", "Item C", "Item D"}."Item C"  # U8
      w526 = "\"Item C\""
      n243 = call "JSON Flatten.vi"("Enums as string? (F)"=TRUE, "error in (no error)"=w533, "Variant in"=w525) -> ("error out"=w534:errorcluster, "JSON out"=w531:string)  [unwired: 7 in]
      n244 = call "JSON Unflatten.vi"("Variant Type"=w524, "error in (no error)"=w534, "JSON in"=w531) -> ("error out"=w532:errorcluster, "Exists?"=w529:bool, "Variant out"=w530:variant)  [unwired: 6 in]
      n245 = Variant To Data(error in=w532, type=w524, Variant=w530) -> (data=w528:enum8{"Item A", "Item B", "Item C", "Item D"}, error out=w522:errorcluster)
      n246 = Equal?(x=w525, y=w528) -> (x = y?=w527:bool)
      n247 = Equal?(x=w526, y=w531) -> (x = y?=w537:bool)
      n248 = To Variant(anything=w528) -> (Variant=w535:variant)
      n249 = Compound Arithmetic op=AND(w537, w529, w527, invert w522) -> (w536:bool)
    }
    frame "EnumBadString" {
      w541 = enum16{"Item A", "Item B", "Item C", "Item D"}."Item A"  # U16
      w542 = T3."Item E"  # U16
      w543 = "\"Item E\""
      n250 = call "JSON Flatten.vi"("Enums as string? (F)"=TRUE, "error in (no error)"=w549, "Variant in"=w542) -> ("error out"=w550:errorcluster, "JSON out"=w547:string)  [unwired: 7 in]
      n251 = call "JSON Unflatten.vi"("Variant Type"=w541, "error in (no error)"=w550, "JSON in"=w547) -> ("error out"=w548:errorcluster, "Exists?"=w545:bool, "Variant out"=w546:variant)  [unwired: 6 in]
      n252 = Variant To Data(error in=w548, type=w541, Variant=w546) -> (data=w544:enum16{"Item A", "Item B", "Item C", "Item D"}, error out=w538:errorcluster)
      n253 = Equal?(x=w543, y=w547) -> (x = y?=w553:bool)
      n254 = To Variant(anything=w544) -> (Variant=w551:variant)
      n255 = call <vilib>:"Clear Errors.vi"("error in (no error)"=w538) -> ("error out"=w539:errorcluster)  [unwired: 5 in, 1 out]
      n256 = Compound Arithmetic op=AND(w553, invert w545, w538) -> (w552:bool)
    }
    frame "PathAbs" {
      w555 = path ""
      w556 = path "C:/"
      w557 = "\"C:\\\\\""
      n257 = call "JSON Flatten.vi"("error in (no error)"=w564, "Variant in"=w556) -> ("error out"=w565:errorcluster, "JSON out"=w562:string)  [unwired: 8 in]
      n258 = call "JSON Unflatten.vi"("Variant Type"=w555, "error in (no error)"=w565, "JSON in"=w562) -> ("error out"=w563:errorcluster, "Exists?"=w560:bool, "Variant out"=w561:variant)  [unwired: 6 in]
      n259 = Variant To Data(error in=w563, type=w555, Variant=w561) -> (data=w559:path, error out=w554:errorcluster)
      n260 = Equal?(x=w556, y=w559) -> (x = y?=w558:bool)
      n261 = Equal?(x=w557, y=w562) -> (x = y?=w568:bool)
      n262 = To Variant(anything=w559) -> (Variant=w566:variant)
      n263 = Compound Arithmetic op=AND(w568, w560, w558, invert w554) -> (w567:bool)
    }
    frame "PathRel" {
      w570 = path ""
      w571 = path "abc/def.txt"
      w572 = "\"abc\\\\def.txt\""
      n264 = call "JSON Flatten.vi"("error in (no error)"=w579, "Variant in"=w571) -> ("error out"=w580:errorcluster, "JSON out"=w577:string)  [unwired: 8 in]
      n265 = call "JSON Unflatten.vi"("Variant Type"=w570, "error in (no error)"=w580, "JSON in"=w577) -> ("error out"=w578:errorcluster, "Exists?"=w575:bool, "Variant out"=w576:variant)  [unwired: 6 in]
      n266 = Variant To Data(error in=w578, type=w570, Variant=w576) -> (data=w574:path, error out=w569:errorcluster)
      n267 = Equal?(x=w571, y=w574) -> (x = y?=w573:bool)
      n268 = Equal?(x=w572, y=w577) -> (x = y?=w583:bool)
      n269 = To Variant(anything=w574) -> (Variant=w581:variant)
      n270 = Compound Arithmetic op=AND(w583, w575, w573, invert w569) -> (w582:bool)
    }
    frame "PathNetwork" {
      w585 = path ""
      w586 = path "\\\\server\\folder"
      w587 = "\"\\\\\\\\server\\\\folder\""
      n271 = call "JSON Flatten.vi"("error in (no error)"=w594, "Variant in"=w586) -> ("error out"=w595:errorcluster, "JSON out"=w592:string)  [unwired: 8 in]
      n272 = call "JSON Unflatten.vi"("Variant Type"=w585, "error in (no error)"=w595, "JSON in"=w592) -> ("error out"=w593:errorcluster, "Exists?"=w590:bool, "Variant out"=w591:variant)  [unwired: 6 in]
      n273 = Variant To Data(error in=w593, type=w585, Variant=w591) -> (data=w589:path, error out=w584:errorcluster)
      n274 = Equal?(x=w586, y=w589) -> (x = y?=w588:bool)
      n275 = Equal?(x=w587, y=w592) -> (x = y?=w598:bool)
      n276 = To Variant(anything=w589) -> (Variant=w596:variant)
      n277 = Compound Arithmetic op=AND(w598, w590, w588, invert w584) -> (w597:bool)
    }
    frame "PathFile" {
      w600 = path ""
      w601 = path "file.txt"
      w602 = "\"file.txt\""
      n278 = call "JSON Flatten.vi"("error in (no error)"=w609, "Variant in"=w601) -> ("error out"=w610:errorcluster, "JSON out"=w607:string)  [unwired: 8 in]
      n279 = call "JSON Unflatten.vi"("Variant Type"=w600, "error in (no error)"=w610, "JSON in"=w607) -> ("error out"=w608:errorcluster, "Exists?"=w605:bool, "Variant out"=w606:variant)  [unwired: 6 in]
      n280 = Variant To Data(error in=w608, type=w600, Variant=w606) -> (data=w604:path, error out=w599:errorcluster)
      n281 = Equal?(x=w601, y=w604) -> (x = y?=w603:bool)
      n282 = Equal?(x=w602, y=w607) -> (x = y?=w613:bool)
      n283 = To Variant(anything=w604) -> (Variant=w611:variant)
      n284 = Compound Arithmetic op=AND(w613, w605, w603, invert w599) -> (w612:bool)
    }
    frame "PathEmpty" {
      w615 = path ""
      w616 = path ""
      w617 = "\"\""
      n285 = call "JSON Flatten.vi"("error in (no error)"=w624, "Variant in"=w615) -> ("error out"=w625:errorcluster, "JSON out"=w622:string)  [unwired: 8 in]
      n286 = call "JSON Unflatten.vi"("Variant Type"=w616, "error in (no error)"=w625, "JSON in"=w622) -> ("error out"=w623:errorcluster, "Exists?"=w620:bool, "Variant out"=w621:variant)  [unwired: 6 in]
      n287 = Variant To Data(error in=w623, type=w616, Variant=w621) -> (data=w619:path, error out=w614:errorcluster)
      n288 = Equal?(x=w615, y=w619) -> (x = y?=w618:bool)
      n289 = Equal?(x=w617, y=w622) -> (x = y?=w628:bool)
      n290 = To Variant(anything=w619) -> (Variant=w626:variant)
      n291 = Compound Arithmetic op=AND(w628, w620, w618, invert w614) -> (w627:bool)
    }
    frame "PathNaN" {
      w630 = path ""
      w631 = path ""
      w632 = "null"
      n292 = call "JSON Flatten.vi"("error in (no error)"=w639, "Variant in"=w630) -> ("error out"=w640:errorcluster, "JSON out"=w637:string)  [unwired: 8 in]
      n293 = call "JSON Unflatten.vi"("Variant Type"=w631, "error in (no error)"=w640, "JSON in"=w637) -> ("error out"=w638:errorcluster, "Exists?"=w635:bool, "Variant out"=w636:variant)  [unwired: 6 in]
      n294 = Variant To Data(error in=w638, type=w631, Variant=w636) -> (data=w634:path, error out=w629:errorcluster)
      n295 = Equal?(x=w630, y=w634) -> (x = y?=w633:bool)
      n296 = Equal?(x=w632, y=w637) -> (x = y?=w643:bool)
      n297 = To Variant(anything=w634) -> (Variant=w641:variant)
      n298 = Compound Arithmetic op=AND(w643, w635, w633, invert w629) -> (w642:bool)
    }
    frame "PathCurrentDir" {
      w645 = path ""
      w646 = path ""
      w647 = "\".\""
      n299 = call "JSON Flatten.vi"("error in (no error)"=w654, "Variant in"=w645) -> ("error out"=w655:errorcluster, "JSON out"=w652:string)  [unwired: 8 in]
      n300 = call "JSON Unflatten.vi"("Variant Type"=w646, "error in (no error)"=w655, "JSON in"=w652) -> ("error out"=w653:errorcluster, "Exists?"=w650:bool, "Variant out"=w651:variant)  [unwired: 6 in]
      n301 = Variant To Data(error in=w653, type=w646, Variant=w651) -> (data=w649:path, error out=w644:errorcluster)
      n302 = Equal?(x=w645, y=w649) -> (x = y?=w648:bool)
      n303 = Equal?(x=w647, y=w652) -> (x = y?=w658:bool)
      n304 = To Variant(anything=w649) -> (Variant=w656:variant)
      n305 = Compound Arithmetic op=AND(w658, w650, w648, invert w644) -> (w657:bool)
    }
    frame "PathParentDir" {
      w660 = path ".."
      w661 = path ""
      w662 = "\"..\""
      n306 = call "JSON Flatten.vi"("error in (no error)"=w669, "Variant in"=w660) -> ("error out"=w670:errorcluster, "JSON out"=w667:string)  [unwired: 8 in]
      n307 = call "JSON Unflatten.vi"("Variant Type"=w661, "error in (no error)"=w670, "JSON in"=w667) -> ("error out"=w668:errorcluster, "Exists?"=w665:bool, "Variant out"=w666:variant)  [unwired: 6 in]
      n308 = Variant To Data(error in=w668, type=w661, Variant=w666) -> (data=w664:path, error out=w659:errorcluster)
      n309 = Equal?(x=w660, y=w664) -> (x = y?=w663:bool)
      n310 = Equal?(x=w662, y=w667) -> (x = y?=w673:bool)
      n311 = To Variant(anything=w664) -> (Variant=w671:variant)
      n312 = Compound Arithmetic op=AND(w673, w665, w663, invert w659) -> (w672:bool)
    }
    frame "TimeDateTime" {
      w683 = ext 1e-13  # EXT
      w687 = timestamp(0 s since 1904-01-01)
      w679 = timestamp(3677191673.3029866 s since 1904-01-01) ("Time Stamp")
      # "ISO8601"
      n313 = call "JSON Flatten.vi"("error in (no error)"=w694, "Variant in"=w679) -> ("error out"=w695:errorcluster, "JSON out"=w692:string)  [unwired: 8 in]
      n314 = call "JSON Timestamp to ISO8601.vi"("To UTC? (F)"=FALSE, "Local Date Time"=w679) -> ("ISO 8601 Date Time"=w677:string)  [unwired: 9 in]
      n315 = call "JSON Unflatten.vi"("Variant Type"=w687, "error in (no error)"=w695, "JSON in"=w692) -> ("error out"=w693:errorcluster, "Exists?"=w690:bool, "Variant out"=w691:variant)  [unwired: 6 in]
      n316 = Concatenate Strings("\"" ("string"), w677, "\"" ("string")) -> (w676:string)
      n317 = Variant To Data(error in=w693, type=w687, Variant=w691) -> (data=w689:timestamp, error out=w688:errorcluster)
      n318 = To Extended Precision Float(1:w679) -> (0:w682:ext)
      n319 = To Extended Precision Float(1:w689) -> (0:w681:ext)
      n320 = Subtract(x=w682, y=w681) -> (x-y=w686:ext)
      n321 = Equal?(x=w676, y=w692) -> (x = y?=w698:bool)
      n322 = Absolute Value(x=w686) -> (abs(x)=w685:ext)
      n323 = Divide(x=w685, y=w681) -> (x/y=w684:ext)
      n324 = Less Or Equal?(x=w684, y=w683) -> (x <= y?=w680:bool)
      n325 = To Variant(anything=w689) -> (Variant=w696:variant)
      n326 = Compound Arithmetic op=AND(w698, w690, w680, invert w688) -> (w697:bool)
    }
    frame "TimeDate" {
      w700 = "2020-11-13" ("JSON in")
      w708 = ext 1e-13  # EXT
      w712 = timestamp(0 s since 1904-01-01)
      # "ISO8601"
      n327 = call "JSON ISO8601 to Timestamp.vi"("ISO 8601 Date Time"=w700) -> ("Local Time Stamp"=w701:timestamp)  [unwired: 10 in]
      n328 = Concatenate Strings("\"" ("string"), w700, "\"" ("string")) -> (w699:string)
      n329 = call "JSON Unflatten.vi"("Variant Type"=w712, "error in (no error)"=w702, "JSON in"=w699) -> ("error out"=w717:errorcluster, "Exists?"=w715:bool, "Variant out"=w716:variant)  [unwired: 6 in]
      n330 = Variant To Data(error in=w717, type=w712, Variant=w716) -> (data=w714:timestamp, error out=w713:errorcluster)
      n331 = To Extended Precision Float(1:w701) -> (0:w707:ext)
      n332 = To Extended Precision Float(1:w714) -> (0:w706:ext)
      n333 = Subtract(x=w707, y=w706) -> (x-y=w711:ext)
      n334 = Equal?(x=w699, y=w699) -> (x = y?=w720:bool)
      n335 = Absolute Value(x=w711) -> (abs(x)=w710:ext)
      n336 = Divide(x=w710, y=w706) -> (x/y=w709:ext)
      n337 = Less Or Equal?(x=w709, y=w708) -> (x <= y?=w705:bool)
      n338 = To Variant(anything=w714) -> (Variant=w718:variant)
      n339 = Compound Arithmetic op=AND(w720, w715, w705, invert w713) -> (w719:bool)
    }
    frame "NullVoid" {
      w724 = variant
      w728 = "null"
      # "Variant to Data on void\ncauses error 1"
      n340 = call "JSON Flatten.vi"("error in (no error)"=w731, "Variant in"=w724) -> ("error out"=w732:errorcluster, "JSON out"=w730:string)  [unwired: 8 in]
      n341 = call "JSON Unflatten.vi"("Variant Type"=variant, "error in (no error)"=w732, "JSON in"=w730) -> ("error out"=w725:errorcluster, "Exists?"=w729:bool, "Variant out"=w723:variant)  [unwired: 6 in]
      n342 = Variant To Flattened String(Variant=w724) -> (data string=w722:string)  [unwired: 1 out]
      n343 = Variant To Flattened String(Variant=w723) -> (data string=w721:string)  [unwired: 1 out]
      n344 = Equal?(x=w722, y=w721) -> (x = y?=w727:bool)
      n345 = Equal?(x=w728, y=w730) -> (x = y?=w735:bool)
      n346 = To Variant(anything=w723) -> (Variant=w733:variant)
      n347 = Compound Arithmetic op=AND(w735, w729, w727, invert w725) -> (w734:bool)
    }
    frame "NullLVVariant" {
      w737 = variant
      w736 = variant
      w747 = "null"
      n348 = To Variant(anything=w736) -> (Variant=w742:variant)
      n349 = call "JSON Flatten.vi"("error in (no error)"=w750, "Variant in"=w742) -> ("error out"=w751:errorcluster, "JSON out"=w749:string)  [unwired: 8 in]
      n350 = To Variant(anything=w737) -> (Variant=w741:variant)
      n351 = call "JSON Unflatten.vi"("Variant Type"=w741, "error in (no error)"=w751, "JSON in"=w749) -> ("error out"=w745:errorcluster, "Exists?"=w748:bool, "Variant out"=w739:variant)  [unwired: 6 in]
      n352 = Variant To Data(error in=w745, type=w737, Variant=w739) -> (data=w738:variant, error out=w740:errorcluster)
      n353 = Variant To Flattened String(Variant=w736) -> (data string=w744:string)  [unwired: 1 out]
      n354 = Variant To Flattened String(Variant=w738) -> (data string=w743:string)  [unwired: 1 out]
      n355 = Equal?(x=w744, y=w743) -> (x = y?=w746:bool)
      n356 = Equal?(x=w747, y=w749) -> (x = y?=w754:bool)
      n357 = To Variant(anything=w738) -> (Variant=w752:variant)
      n358 = Compound Arithmetic op=AND(w754, w748, w746, invert w740) -> (w753:bool)
    }
    frame "NullBoolean" {
      w757 = TRUE
      w755 = "null"
      n359 = call "JSON Unflatten.vi"("Variant Type"=w757, "error in (no error)"=w758, "JSON in"=w755) -> ("error out"=w762:errorcluster, "Exists?"=w760:bool, "Variant out"=w761:variant)  [unwired: 6 in]
      n360 = Variant To Data(error in=w762, type=w757, Variant=w761) -> (data=w756:bool, error out=w759:errorcluster)
      n361 = Equal?(x=w755, y=w755) -> (x = y?=w765:bool)
      n362 = To Variant(anything=w756) -> (Variant=w763:variant)
      n363 = Compound Arithmetic op=AND(w765, w760, invert w756, invert w759) -> (w764:bool)
    }
    frame "NullInt" {
      w767 = 0  # I32
      w769 = -1  # I32
      w770 = "null"
      n364 = call "JSON Unflatten.vi"("Variant Type"=w769, "error in (no error)"=w771, "JSON in"=w770) -> ("error out"=w775:errorcluster, "Exists?"=w773:bool, "Variant out"=w774:variant)  [unwired: 6 in]
      n365 = Variant To Data(error in=w775, type=w769, Variant=w774) -> (data=w768:i32, error out=w772:errorcluster)
      n366 = Equal?(x=w767, y=w768) -> (x = y?=w766:bool)
      n367 = Equal?(x=w770, y=w770) -> (x = y?=w778:bool)
      n368 = To Variant(anything=w768) -> (Variant=w776:variant)
      n369 = Compound Arithmetic op=AND(w778, w773, w766, invert w772) -> (w777:bool)
    }
    frame "NullUint" {
      w780 = u32 0  # U32
      w782 = u32 1  # U32
      w783 = "null"
      n370 = call "JSON Unflatten.vi"("Variant Type"=w782, "error in (no error)"=w784, "JSON in"=w783) -> ("error out"=w788:errorcluster, "Exists?"=w786:bool, "Variant out"=w787:variant)  [unwired: 6 in]
      n371 = Variant To Data(error in=w788, type=w782, Variant=w787) -> (data=w781:u32, error out=w785:errorcluster)
      n372 = Equal?(x=w780, y=w781) -> (x = y?=w779:bool)
      n373 = Equal?(x=w783, y=w783) -> (x = y?=w791:bool)
      n374 = To Variant(anything=w781) -> (Variant=w789:variant)
      n375 = Compound Arithmetic op=AND(w791, w786, w779, invert w785) -> (w790:bool)
    }
    frame "NullFloat" {
      w793 = 0.0  # DBL
      w795 = 1.0  # DBL
      w796 = "null"
      n376 = call "JSON Unflatten.vi"("Variant Type"=w795, "error in (no error)"=w797, "JSON in"=w796) -> ("error out"=w801:errorcluster, "Exists?"=w799:bool, "Variant out"=w800:variant)  [unwired: 6 in]
      n377 = Variant To Data(error in=w801, type=w795, Variant=w800) -> (data=w794:dbl, error out=w798:errorcluster)
      n378 = Equal?(x=w793, y=w794) -> (x = y?=w792:bool)
      n379 = Equal?(x=w796, y=w796) -> (x = y?=w804:bool)
      n380 = To Variant(anything=w794) -> (Variant=w802:variant)
      n381 = Compound Arithmetic op=AND(w804, w799, w792, invert w798) -> (w803:bool)
    }
    frame "NullString" {
      w808 = "x"
      w809 = "null"
      n382 = call "JSON Unflatten.vi"("Variant Type"=w808, "error in (no error)"=w810, "JSON in"=w809) -> ("error out"=w814:errorcluster, "Exists?"=w812:bool, "Variant out"=w813:variant)  [unwired: 6 in]
      n383 = Variant To Data(error in=w814, type=w808, Variant=w813) -> (data=w807:string, error out=w811:errorcluster)
      n384 = Equal?(x="", y=w807) -> (x = y?=w805:bool)
      n385 = Equal?(x=w809, y=w809) -> (x = y?=w817:bool)
      n386 = To Variant(anything=w807) -> (Variant=w815:variant)
      n387 = Compound Arithmetic op=AND(w817, w812, w805, invert w811) -> (w816:bool)
    }
    frame "NullPath" {
      w820 = path "C:/"
      w821 = "null"
      n388 = call "JSON Unflatten.vi"("Variant Type"=w820, "error in (no error)"=w822, "JSON in"=w821) -> ("error out"=w826:errorcluster, "Exists?"=w824:bool, "Variant out"=w825:variant)  [unwired: 6 in]
      n389 = Variant To Data(error in=w826, type=w820, Variant=w825) -> (data=w819:path, error out=w823:errorcluster)
      n390 = Not A Number/Path/Refnum?(number/path/refnum=w819) -> (NaN/Path/Refnum?=w818:bool)
      n391 = Equal?(x=w821, y=w821) -> (x = y?=w829:bool)
      n392 = To Variant(anything=w819) -> (Variant=w827:variant)
      n393 = Compound Arithmetic op=AND(w829, w824, w818, invert w823) -> (w828:bool)
    }
    frame "NullEnum" {
      w831 = enum16{"Item A", "Item B", "Item C"}."Item B"
      w834 = "null"
      n394 = call "JSON Unflatten.vi"("Variant Type"=w831, "error in (no error)"=w835, "JSON in"=w834) -> ("error out"=w839:errorcluster, "Exists?"=w837:bool, "Variant out"=w838:variant)  [unwired: 6 in]
      n395 = Variant To Data(error in=w839, type=w831, Variant=w838) -> (data=w833:enum16{"Item A", "Item B", "Item C"}, error out=w836:errorcluster)
      n396 = Equal?(x=enum16{"Item A", "Item B", "Item C"}."Item A", y=w833) -> (x = y?=w832:bool)
      n397 = Equal?(x=w834, y=w834) -> (x = y?=w842:bool)
      n398 = To Variant(anything=w833) -> (Variant=w840:variant)
      n399 = Compound Arithmetic op=AND(w842, w837, w832, invert w836) -> (w841:bool)
    }
    frame "NullTime" {
      w844 = timestamp(3688247390.302975 s since 1904-01-01) ("Time Stamp")
      w847 = "null"
      n400 = call "JSON Unflatten.vi"("Variant Type"=w844, "error in (no error)"=w848, "JSON in"=w847) -> ("error out"=w852:errorcluster, "Exists?"=w850:bool, "Variant out"=w851:variant)  [unwired: 6 in]
      n401 = Variant To Data(error in=w852, type=w844, Variant=w851) -> (data=w846:timestamp, error out=w849:errorcluster)
      n402 = Equal?(x=timestamp(0 s since 1904-01-01), y=w846) -> (x = y?=w845:bool)
      n403 = Equal?(x=w847, y=w847) -> (x = y?=w855:bool)
      n404 = To Variant(anything=w846) -> (Variant=w853:variant)
      n405 = Compound Arithmetic op=AND(w855, w850, w845, invert w849) -> (w854:bool)
    }
    frame "NullArray" {
      w858 = string[] ["a"]
      w861 = "null"
      n406 = call "JSON Unflatten.vi"("Variant Type"=w858, "error in (no error)"=w862, "JSON in"=w861) -> ("error out"=w866:errorcluster, "Exists?"=w864:bool, "Variant out"=w865:variant)  [unwired: 6 in]
      n407 = Variant To Data(error in=w866, type=w858, Variant=w865) -> (data=w860:string[], error out=w863:errorcluster)
      n408 = Equal?(x=string[] [], y=w860) -> (x = y?=w859:bool[])
      n409 = And Array Elements(Boolean array=w859) -> (logical AND=w856:bool)
      n410 = Equal?(x=w861, y=w861) -> (x = y?=w869:bool)
      n411 = To Variant(anything=w860) -> (Variant=w867:variant)
      n412 = Compound Arithmetic op=AND(w869, w864, w856, invert w863) -> (w868:bool)
    }
    frame "NullArrayVoid" {
      w872 = variant[] []
      w874 = "null"
      n413 = call "JSON Unflatten.vi"("Variant Type"=w872, "error in (no error)"=w873, "JSON in"=w874) -> ("error out"=w878:errorcluster, "Exists?"=w876:bool, "Variant out"=w877:variant)  [unwired: 6 in]
      n414 = Variant To Data(error in=w878, type=w872, Variant=w877) -> (data=w871:variant[], error out=w875:errorcluster)
      n415 = Empty Array?(array=w871) -> (empty?=w870:bool)
      n416 = Equal?(x=w874, y=w874) -> (x = y?=w881:bool)
      n417 = To Variant(anything=w871) -> (Variant=w879:variant)
      n418 = Compound Arithmetic op=AND(w881, w876, w870, invert w875) -> (w880:bool)
    }
    frame "NullArrayLVVariant" {
      w888 = "null"
      n419 = To Variant(anything=variant) -> (Variant=w883:variant)
      n420 = Build Array(w883) -> (w882:variant[])
      n421 = call "JSON Unflatten.vi"("Variant Type"=w882, "error in (no error)"=w887, "JSON in"=w888) -> ("error out"=w892:errorcluster, "Exists?"=w890:bool, "Variant out"=w891:variant)  [unwired: 6 in]
      n422 = Variant To Data(error in=w892, type=w882, Variant=w891) -> (data=w886:variant[], error out=w889:errorcluster)
      n423 = Empty Array?(array=w886) -> (empty?=w885:bool)
      n424 = Equal?(x=w888, y=w888) -> (x = y?=w895:bool)
      n425 = To Variant(anything=w886) -> (Variant=w893:variant)
      n426 = Compound Arithmetic op=AND(w895, w890, w885, invert w889) -> (w894:bool)
    }
    frame "NullObject" {
      w898 = T2 {"I16"=1, "Bool"=TRUE, "String"="a", "Array"=[1]} ("Cluster")
      w900 = "null"
      n427 = call "JSON Unflatten.vi"("Variant Type"=w898, "error in (no error)"=w901, "JSON in"=w900) -> ("error out"=w905:errorcluster, "Exists?"=w903:bool, "Variant out"=w904:variant)  [unwired: 6 in]
      n428 = Variant To Data(error in=w905, type=w898, Variant=w904) -> (data=w899:T2, error out=w902:errorcluster)
      n429 = Equal?(x=T2 {"I16"=0, "Bool"=FALSE, "String"="", "Array"=[]} ("Cluster"), y=w899) -> (x = y?=w896:bool)
      n430 = Equal?(x=w900, y=w900) -> (x = y?=w908:bool)
      n431 = To Variant(anything=w899) -> (Variant=w906:variant)
      n432 = Compound Arithmetic op=AND(w908, w903, w896, invert w902) -> (w907:bool)
    }
    frame "NullObjectVoid" {
      w910 = cluster{variant} {variant}
      w913 = "null"
      n433 = call "JSON Unflatten.vi"("Variant Type"=w910, "error in (no error)"=w914, "JSON in"=w913) -> ("error out"=w918:errorcluster, "Exists?"=w916:bool, "Variant out"=w917:variant)  [unwired: 6 in]
      n434 = Variant To Data(error in=w918, type=w910, Variant=w917) -> (data=w912:cluster{variant}, error out=w915:errorcluster)
      n435 = Equal?(x=cluster{variant} {variant}, y=w912) -> (x = y?=w911:bool)
      n436 = Equal?(x=w913, y=w913) -> (x = y?=w921:bool)
      n437 = To Variant(anything=w912) -> (Variant=w919:variant)
      n438 = Compound Arithmetic op=AND(w921, w916, w911, invert w915) -> (w920:bool)
    }
    frame "NullObjectLVVariant" {
      w923 = variant
      w928 = "null"
      n439 = To Variant(anything=w923) -> (Variant=w926:variant)
      n440 = Bundle("Variant"=w926) -> (w925:cluster{"Variant":variant})  [unwired: 1 in]
      n441 = call "JSON Unflatten.vi"("Variant Type"=w925, "error in (no error)"=w929, "JSON in"=w928) -> ("error out"=w933:errorcluster, "Exists?"=w931:bool, "Variant out"=w932:variant)  [unwired: 6 in]
      n442 = Variant To Data(error in=w933, type=w925, Variant=w932) -> (data=w924:cluster{"Variant":variant}, error out=w930:errorcluster)
      n443 = Unbundle By Name(w924) -> ("Variant"=w922:variant)
      n444 = Equal?(x=w923, y=w922) -> (x = y?=w927:bool)
      n445 = Equal?(x=w928, y=w928) -> (x = y?=w936:bool)
      n446 = To Variant(anything=w924) -> (Variant=w934:variant)
      n447 = Compound Arithmetic op=AND(w936, w931, w927, invert w930) -> (w935:bool)
    }
    frame "NullWaveform" {
      w938 = waveform(dbl) {"t0"=timestamp(3681289404.123456 s since 1904-01-01), "dt"=0.5, "Y"=[1.1, 2.2, 3.3]} ("Waveform")
      w941 = "null"
      n448 = call "JSON Unflatten.vi"("Variant Type"=w938, "error in (no error)"=w942, "JSON in"=w941) -> ("error out"=w946:errorcluster, "Exists?"=w944:bool, "Variant out"=w945:variant)  [unwired: 6 in]
      n449 = Variant To Data(error in=w946, type=w938, Variant=w945) -> (data=w940:waveform(dbl), error out=w943:errorcluster)
      n450 = Equal?(x=waveform(dbl) {"t0"=timestamp(0 s since 1904-01-01), "dt"=0.0, "Y"=[]} ("Waveform"), y=w940) -> (x = y?=w939:bool)
      n451 = Equal?(x=w941, y=w941) -> (x = y?=w949:bool)
      n452 = To Variant(anything=w940) -> (Variant=w947:variant)
      n453 = Compound Arithmetic op=AND(w949, w944, w939, invert w943) -> (w948:bool)
    }
    frame "Array1DValues" {
      w952 = i32[] []  # I32
      w953 = i32[] [1, 2, 3]  # I32
      w954 = "[1,2,3]"
      n454 = call "JSON Flatten.vi"("error in (no error)"=w961, "Variant in"=w953) -> ("error out"=w962:errorcluster, "JSON out"=w959:string)  [unwired: 8 in]
      n455 = call "JSON Unflatten.vi"("Variant Type"=w952, "error in (no error)"=w962, "JSON in"=w959) -> ("error out"=w960:errorcluster, "Exists?"=w957:bool, "Variant out"=w958:variant)  [unwired: 6 in]
      n456 = Variant To Data(error in=w960, type=w952, Variant=w958) -> (data=w956:i32[], error out=w951:errorcluster)
      n457 = Equal?(x=w953, y=w956) -> (x = y?=w955:bool[])
      n458 = And Array Elements(Boolean array=w955) -> (logical AND=w950:bool)
      n459 = Equal?(x=w954, y=w959) -> (x = y?=w965:bool)
      n460 = To Variant(anything=w956) -> (Variant=w963:variant)
      n461 = Compound Arithmetic op=AND(w965, w957, w950, invert w951) -> (w964:bool)
    }
    frame "Array1DEmpty" {
      w968 = i32[] [1]  # I32
      w969 = i32[] []  # I32
      w970 = "[]"
      n462 = call "JSON Flatten.vi"("error in (no error)"=w977, "Variant in"=w969) -> ("error out"=w978:errorcluster, "JSON out"=w975:string)  [unwired: 8 in]
      n463 = call "JSON Unflatten.vi"("Variant Type"=w968, "error in (no error)"=w978, "JSON in"=w975) -> ("error out"=w976:errorcluster, "Exists?"=w973:bool, "Variant out"=w974:variant)  [unwired: 6 in]
      n464 = Variant To Data(error in=w976, type=w968, Variant=w974) -> (data=w972:i32[], error out=w967:errorcluster)
      n465 = Equal?(x=w969, y=w972) -> (x = y?=w971:bool[])
      n466 = And Array Elements(Boolean array=w971) -> (logical AND=w966:bool)
      n467 = Equal?(x=w970, y=w975) -> (x = y?=w981:bool)
      n468 = To Variant(anything=w972) -> (Variant=w979:variant)
      n469 = Compound Arithmetic op=AND(w981, w973, w966, invert w967) -> (w980:bool)
    }
    frame "Array1DObject" {
      w983 = errorcluster[] []
      w984 = "[{\"status\":true,\"code\":8,\"source\":\"abc\"},{\"status\":false,\"code\":9,\"source\":\"def\"},{\"status\":true,\"code\":10,\"source\":\"ghi\"}]"
      w985 = errorcluster[] [{"status"=TRUE, "code"=8, "source"="abc"}, {"status"=FALSE, "code"=9, "source"="def"}, {"status"=TRUE, "code"=10, "source"="ghi"}]
      n470 = call "JSON Flatten.vi"("error in (no error)"=w992, "Variant in"=w985) -> ("error out"=w993:errorcluster, "JSON out"=w990:string)  [unwired: 8 in]
      n471 = call "JSON Unflatten.vi"("Variant Type"=w983, "error in (no error)"=w993, "JSON in"=w990) -> ("error out"=w991:errorcluster, "Exists?"=w988:bool, "Variant out"=w989:variant)  [unwired: 6 in]
      n472 = Variant To Data(error in=w991, type=w983, Variant=w989) -> (data=w987:errorcluster[], error out=w986:errorcluster)
      n473 = Equal?(x=w985, y=w987) -> (x = y?=w982:bool)
      n474 = Equal?(x=w984, y=w990) -> (x = y?=w996:bool)
      n475 = To Variant(anything=w987) -> (Variant=w994:variant)
      n476 = Compound Arithmetic op=AND(w996, w988, w982, invert w986) -> (w995:bool)
    }
    frame "Array1DMulti" {
      w1018 = "[true,3,\"abc\",{\"status\":true,\"code\":10,\"source\":\"ghi\"}]"
      # "Note: Multityped array data must be built into the variant array\nso that the variant type definitions can parse the data successfully"
      n477 = To Variant(anything=FALSE) -> (Variant=w1002:variant)
      n478 = To Variant(anything=u64 0) -> (Variant=w1004:variant)
      n479 = To Variant(anything="") -> (Variant=w1006:variant)
      n480 = To Variant(anything=errorcluster {"status"=FALSE, "code"=0, "source"=""} ("error out")) -> (Variant=w1008:variant)
      n481 = To Variant(anything=TRUE) -> (Variant=w1016:variant)
      n482 = To Variant(anything=u64 3) -> (Variant=w1014:variant)
      n483 = To Variant(anything="abc") -> (Variant=w1012:variant)
      n484 = To Variant(anything=errorcluster {"status"=TRUE, "code"=10, "source"="ghi"} ("error out")) -> (Variant=w1010:variant)
      n485 = Build Array(w1002, w1004, w1006, w1008) -> (w1000:variant[])
      n486 = Build Array(w1016, w1014, w1012, w1010) -> (w999:variant[])
      n487 = call "JSON Flatten.vi"("error in (no error)"=w1024, "Variant in"=w999) -> ("error out"=w1025:errorcluster, "JSON out"=w1022:string)  [unwired: 8 in]
      n488 = call "JSON Unflatten.vi"("Variant Type"=w1000, "error in (no error)"=w1025, "JSON in"=w1022) -> ("error out"=w1023:errorcluster, "Exists?"=w1020:bool, "Variant out"=w1021:variant)  [unwired: 6 in]
      n489 = Variant To Data(error in=w1023, type=w1000, Variant=w1021) -> (data=w998:variant[], error out=w1019:errorcluster)
      n490 = Equal?(x=w999, y=w998) -> (x = y?=w997:bool[])
      n491 = Equal?(x=w1018, y=w1022) -> (x = y?=w1028:bool)
      n492 = And Array Elements(Boolean array=w997) -> (logical AND=w1009:bool)
      n493 = To Variant(anything=w998) -> (Variant=w1026:variant)
      n494 = Compound Arithmetic op=AND(w1028, w1020, w1009, invert w1019) -> (w1027:bool)
    }
    frame "Array2DValues" {
      w1031 = i32[][] []  # I32
      w1032 = i32[][] [[1, 2, 3], [4, 5, 6]]  # I32
      w1033 = "[[1,2,3],[4,5,6]]"
      n495 = call "JSON Flatten.vi"("error in (no error)"=w1040, "Variant in"=w1032) -> ("error out"=w1041:errorcluster, "JSON out"=w1038:string)  [unwired: 8 in]
      n496 = call "JSON Unflatten.vi"("Variant Type"=w1031, "error in (no error)"=w1041, "JSON in"=w1038) -> ("error out"=w1039:errorcluster, "Exists?"=w1036:bool, "Variant out"=w1037:variant)  [unwired: 6 in]
      n497 = Variant To Data(error in=w1039, type=w1031, Variant=w1037) -> (data=w1035:i32[][], error out=w1030:errorcluster)
      n498 = Equal?(x=w1032, y=w1035) -> (x = y?=w1034:bool[][])
      n499 = And Array Elements(Boolean array=w1034) -> (logical AND=w1029:bool)
      n500 = Equal?(x=w1033, y=w1038) -> (x = y?=w1044:bool)
      n501 = To Variant(anything=w1035) -> (Variant=w1042:variant)
      n502 = Compound Arithmetic op=AND(w1044, w1036, w1029, invert w1030) -> (w1043:bool)
    }
    frame "Array2DEmpty" {
      w1047 = i32[][] [[1]]  # I32
      w1048 = i32[][] []  # I32
      w1049 = "[]"
      n503 = call "JSON Flatten.vi"("error in (no error)"=w1056, "Variant in"=w1048) -> ("error out"=w1057:errorcluster, "JSON out"=w1054:string)  [unwired: 8 in]
      n504 = call "JSON Unflatten.vi"("Variant Type"=w1047, "error in (no error)"=w1057, "JSON in"=w1054) -> ("error out"=w1055:errorcluster, "Exists?"=w1052:bool, "Variant out"=w1053:variant)  [unwired: 6 in]
      n505 = Variant To Data(error in=w1055, type=w1047, Variant=w1053) -> (data=w1051:i32[][], error out=w1046:errorcluster)
      n506 = Equal?(x=w1048, y=w1051) -> (x = y?=w1050:bool[][])
      n507 = And Array Elements(Boolean array=w1050) -> (logical AND=w1045:bool)
      n508 = Equal?(x=w1049, y=w1054) -> (x = y?=w1060:bool)
      n509 = To Variant(anything=w1051) -> (Variant=w1058:variant)
      n510 = Compound Arithmetic op=AND(w1060, w1052, w1045, invert w1046) -> (w1059:bool)
    }
    frame "Array3DValues" {
      w1063 = i32[][][] []  # I32
      w1064 = i32[][][] [[[1, 2, 3], [4, 5, 6]], [[7, 8, 0], [0, 0, 9]]]  # I32
      w1065 = "[[[1,2,3],[4,5,6]],[[7,8,0],[0,0,9]]]"
      n511 = call "JSON Flatten.vi"("error in (no error)"=w1072, "Variant in"=w1064) -> ("error out"=w1073:errorcluster, "JSON out"=w1070:string)  [unwired: 8 in]
      n512 = call "JSON Unflatten.vi"("Variant Type"=w1063, "error in (no error)"=w1073, "JSON in"=w1070) -> ("error out"=w1071:errorcluster, "Exists?"=w1068:bool, "Variant out"=w1069:variant)  [unwired: 6 in]
      n513 = Variant To Data(error in=w1071, type=w1063, Variant=w1069) -> (data=w1067:i32[][][], error out=w1062:errorcluster)
      n514 = Equal?(x=w1064, y=w1067) -> (x = y?=w1066:bool[][][])
      n515 = And Array Elements(Boolean array=w1066) -> (logical AND=w1061:bool)
      n516 = Equal?(x=w1065, y=w1070) -> (x = y?=w1076:bool)
      n517 = To Variant(anything=w1067) -> (Variant=w1074:variant)
      n518 = Compound Arithmetic op=AND(w1076, w1068, w1061, invert w1062) -> (w1075:bool)
    }
    frame "Array3DEmpty" {
      w1079 = i32[][][] [[[1]]]  # I32
      w1080 = i32[][][] []  # I32
      w1081 = "[]"
      n519 = call "JSON Flatten.vi"("error in (no error)"=w1088, "Variant in"=w1080) -> ("error out"=w1089:errorcluster, "JSON out"=w1086:string)  [unwired: 8 in]
      n520 = call "JSON Unflatten.vi"("Variant Type"=w1079, "error in (no error)"=w1089, "JSON in"=w1086) -> ("error out"=w1087:errorcluster, "Exists?"=w1084:bool, "Variant out"=w1085:variant)  [unwired: 6 in]
      n521 = Variant To Data(error in=w1087, type=w1079, Variant=w1085) -> (data=w1083:i32[][][], error out=w1078:errorcluster)
      n522 = Equal?(x=w1080, y=w1083) -> (x = y?=w1082:bool[][][])
      n523 = And Array Elements(Boolean array=w1082) -> (logical AND=w1077:bool)
      n524 = Equal?(x=w1081, y=w1086) -> (x = y?=w1092:bool)
      n525 = To Variant(anything=w1083) -> (Variant=w1090:variant)
      n526 = Compound Arithmetic op=AND(w1092, w1084, w1077, invert w1078) -> (w1091:bool)
    }
    frame "ObjectValues" {
      w1098 = cluster{"a":i32, "b":string} {"a"=0, "b"=""} ("Cluster")
      w1096 = cluster{"a":i32, "b":string} {"a"=-123, "b"="Hello World"} ("Cluster")
      w1100 = "{\"a\":-123,\"b\":\"Hello World\"}"
      n527 = call "JSON Flatten.vi"("error in (no error)"=w1105, "Variant in"=w1096) -> ("error out"=w1106:errorcluster, "JSON out"=w1103:string)  [unwired: 8 in]
      n528 = call "JSON Unflatten.vi"("Variant Type"=w1098, "error in (no error)"=w1106, "JSON in"=w1103) -> ("error out"=w1104:errorcluster, "Exists?"=w1101:bool, "Variant out"=w1102:variant)  [unwired: 6 in]
      n529 = Variant To Data(error in=w1104, type=w1098, Variant=w1102) -> (data=w1094:cluster{"a":i32, "b":string}, error out=w1099:errorcluster)
      n530 = Variant To Flattened String(Variant=w1096) -> (data string=w1095:string)  [unwired: 1 out]
      n531 = Variant To Flattened String(Variant=w1094) -> (data string=w1093:string)  [unwired: 1 out]
      n532 = Equal?(x=w1095, y=w1093) -> (x = y?=w1097:bool)
      n533 = Equal?(x=w1100, y=w1103) -> (x = y?=w1109:bool)
      n534 = To Variant(anything=w1094) -> (Variant=w1107:variant)
      n535 = Compound Arithmetic op=AND(w1109, w1101, w1097, invert w1099) -> (w1108:bool)
    }
    frame "ObjectEmpty" {
      w1110 = cluster{"null":variant} {"null"=variant} ("Cluster")
      w1114 = cluster{variant} {variant} ("Cluster")
      w1117 = "{}"
      n536 = call "JSON Flatten.vi"("error in (no error)"=w1122, "Variant in"=w1114) -> ("error out"=w1123:errorcluster, "JSON out"=w1120:string)  [unwired: 8 in]
      n537 = call "JSON Unflatten.vi"("Variant Type"=w1110, "error in (no error)"=w1123, "JSON in"=w1120) -> ("error out"=w1121:errorcluster, "Exists?"=w1118:bool, "Variant out"=w1119:variant)  [unwired: 6 in]
      n538 = Variant To Data(error in=w1121, type=w1110, Variant=w1119) -> (data=w1112:cluster{"null":variant}, error out=w1116:errorcluster)
      n539 = Variant To Flattened String(Variant=w1114) -> (data string=w1113:string)  [unwired: 1 out]
      n540 = Variant To Flattened String(Variant=w1112) -> (data string=w1111:string)  [unwired: 1 out]
      n541 = Equal?(x=w1113, y=w1111) -> (x = y?=w1115:bool)
      n542 = Equal?(x=w1117, y=w1120) -> (x = y?=w1126:bool)
      n543 = To Variant(anything=w1112) -> (Variant=w1124:variant)
      n544 = Compound Arithmetic op=AND(w1126, w1118, w1115, invert w1116) -> (w1125:bool)
    }
    frame "ObjectWaveform" {
      w1133 = ext 1e-13  # EXT
      w1155 = waveform(dbl) {"t0"=timestamp(0 s since 1904-01-01), "dt"=1.0, "Y"=[]} ("Waveform")
      w1150 = waveform(dbl) {"t0"=timestamp(3681289404.123456 s since 1904-01-01), "dt"=0.5, "Y"=[1.1, 2.2, 3.3]} ("Waveform")
      n545 = Unbundle By Name(w1150) -> ("t0"=w1154:timestamp)
      n546 = Unbundle By Name(w1150) -> ("t0"=w1149:timestamp, "dt"=w1148:dbl, "Y"=w1147:dbl[])
      n547 = call "JSON Flatten.vi"("error in (no error)"=w1159, "Variant in"=w1150) -> ("error out"=w1160:errorcluster, "JSON out"=w1132:string)  [unwired: 8 in]
      n548 = call "JSON Timestamp to ISO8601.vi"("Local Date Time"=w1154) -> ("ISO 8601 Date Time"=w1153:string)  [unwired: 10 in]
      n549 = To Extended Precision Float(1:w1149) -> (0:w1146:ext)
      n550 = To Extended Precision Float(1:w1148) -> (0:w1145:ext)
      n551 = To Extended Precision Float(1:w1147) -> (0:w1144:ext[])
      n552 = call "JSON Unflatten.vi"("Variant Type"=w1155, "error in (no error)"=w1160, "JSON in"=w1132) -> ("error out"=w1158:errorcluster, "Exists?"=w1130:bool, "Variant out"=w1157:variant)  [unwired: 6 in]
      n553 = Format Into String(format string="{\"t0\":\"%s\",\"dt\":0.5,\"Y\":[1.1,2.2,3.3]}", w1153) -> (resulting string=w1151:string)  [unwired: 2 in, 1 out]
      n554 = Build Array (concatenate)(w1146, w1145, w1144) -> (w1131:ext[])
      n555 = Variant To Data(error in=w1158, type=w1155, Variant=w1157) -> (data=w1137:waveform(dbl), error out=w1156:errorcluster)
      n556 = Unbundle By Name(w1137) -> ("t0"=w1138:timestamp, "dt"=w1139:dbl, "Y"=w1140:dbl[])
      n557 = To Extended Precision Float(1:w1138) -> (0:w1141:ext)
      n558 = To Extended Precision Float(1:w1139) -> (0:w1142:ext)
      n559 = To Extended Precision Float(1:w1140) -> (0:w1143:ext[])
      n560 = Build Array (concatenate)(w1141, w1142, w1143) -> (w1129:ext[])
      n561 = Subtract(x=w1131, y=w1129) -> (x-y=w1136:ext[])
      n562 = Absolute Value(x=w1136) -> (abs(x)=w1135:ext[])
      n563 = Divide(x=w1135, y=w1129) -> (x/y=w1134:ext[])
      n564 = Less Or Equal?(x=w1134, y=w1133) -> (x <= y?=w1128:bool[])
      n565 = And Array Elements(Boolean array=w1128) -> (logical AND=w1127:bool)
      n566 = Equal?(x=w1151, y=w1132) -> (x = y?=w1163:bool)
      n567 = To Variant(anything=w1137) -> (Variant=w1161:variant)
      n568 = Compound Arithmetic op=AND(w1163, w1130, w1127, invert w1156) -> (w1162:bool)
    }
    frame "ObjectReorder" {
      w1172 = cluster{"b":string, "a":i32} {"b"="", "a"=0} ("Cluster")
      w1170 = cluster{"a":i32, "b":string} {"a"=-123, "b"="Hello World"} ("Cluster")
      w1174 = "{\"a\":-123,\"b\":\"Hello World\"}"
      n569 = call "JSON Flatten.vi"("error in (no error)"=w1179, "Variant in"=w1170) -> ("error out"=w1180:errorcluster, "JSON out"=w1177:string)  [unwired: 8 in]
      n570 = call "JSON Unflatten.vi"("Variant Type"=w1172, "error in (no error)"=w1180, "JSON in"=w1177) -> ("error out"=w1178:errorcluster, "Exists?"=w1175:bool, "Variant out"=w1176:variant)  [unwired: 6 in]
      n571 = Variant To Data(error in=w1178, type=w1172, Variant=w1176) -> (data=w1169:cluster{"b":string, "a":i32}, error out=w1173:errorcluster)
      n572 = Unbundle By Name(w1170) -> ("a"=w1168:i32, "b"=w1167:string)
      n573 = Unbundle By Name(w1169) -> ("b"=w1166:string, "a"=w1164:i32)
      n574 = Equal?(x=w1168, y=w1164) -> (x = y?=w1171:bool)
      n575 = Equal?(x=w1167, y=w1166) -> (x = y?=w1165:bool)
      n576 = Equal?(x=w1174, y=w1177) -> (x = y?=w1183:bool)
      n577 = To Variant(anything=w1169) -> (Variant=w1181:variant)
      n578 = Compound Arithmetic op=AND(w1183, w1175, w1171, w1165, invert w1173) -> (w1182:bool)
    }
  }
  "error out" <- w6
  "Passed?" <- w5
  "Result" <- w4
  "JSON in" <- w1
  "JSON out" <- w2
